vi "Auto.vi"() -> ()   [LabVIEW 2020]
uses:
  <vilib>/Utility/miscctls.llb/LVRowAndColumnTypeDef.ctl
  Global_Variable/A131258.vi
  Global_Variable/Global.vi
  Database/Global1.vi
  <userlib>/_MGI/1D Array/MGI Running Average/MGI Running Average(DBL).vi
  <vilib>/addons/database/Connection.llb/DB Tools Open Connec (String).vi
  <vilib>/addons/database/Connection.llb/Conn Execute.vi
  <vilib>/addons/database/Recordset.llb/Rec Fetch Recordset Data (R).vi
  Libraries/S7/S7.lvlib
  <vilib>/addons/database/NI_Database_API.lvlib
panel:
  out "左工位":cluster{dbl[], dbl[]}[](graph)
  in  "判定结果 2":bool[][](array[boolean])=[[TRUE]]
  out "STEP 4":string
  out "STEP 3":string
  in  "STEP 2":string
  out "右code 2":string
  in  "Initialize 7":bool
  in  "Initialize 6":bool
  out "初始化 2":bool[](array[boolean])
  out "左code":string
  out "右工位":cluster{dbl[], dbl[]}[](graph)
  in  "Initialize 4":bool
  in  "Initialize 2":bool
  out "初始化":bool[](array[boolean])
  in  "判定结果":bool[][](array[boolean])=[[TRUE]]
  in  "STEP":string
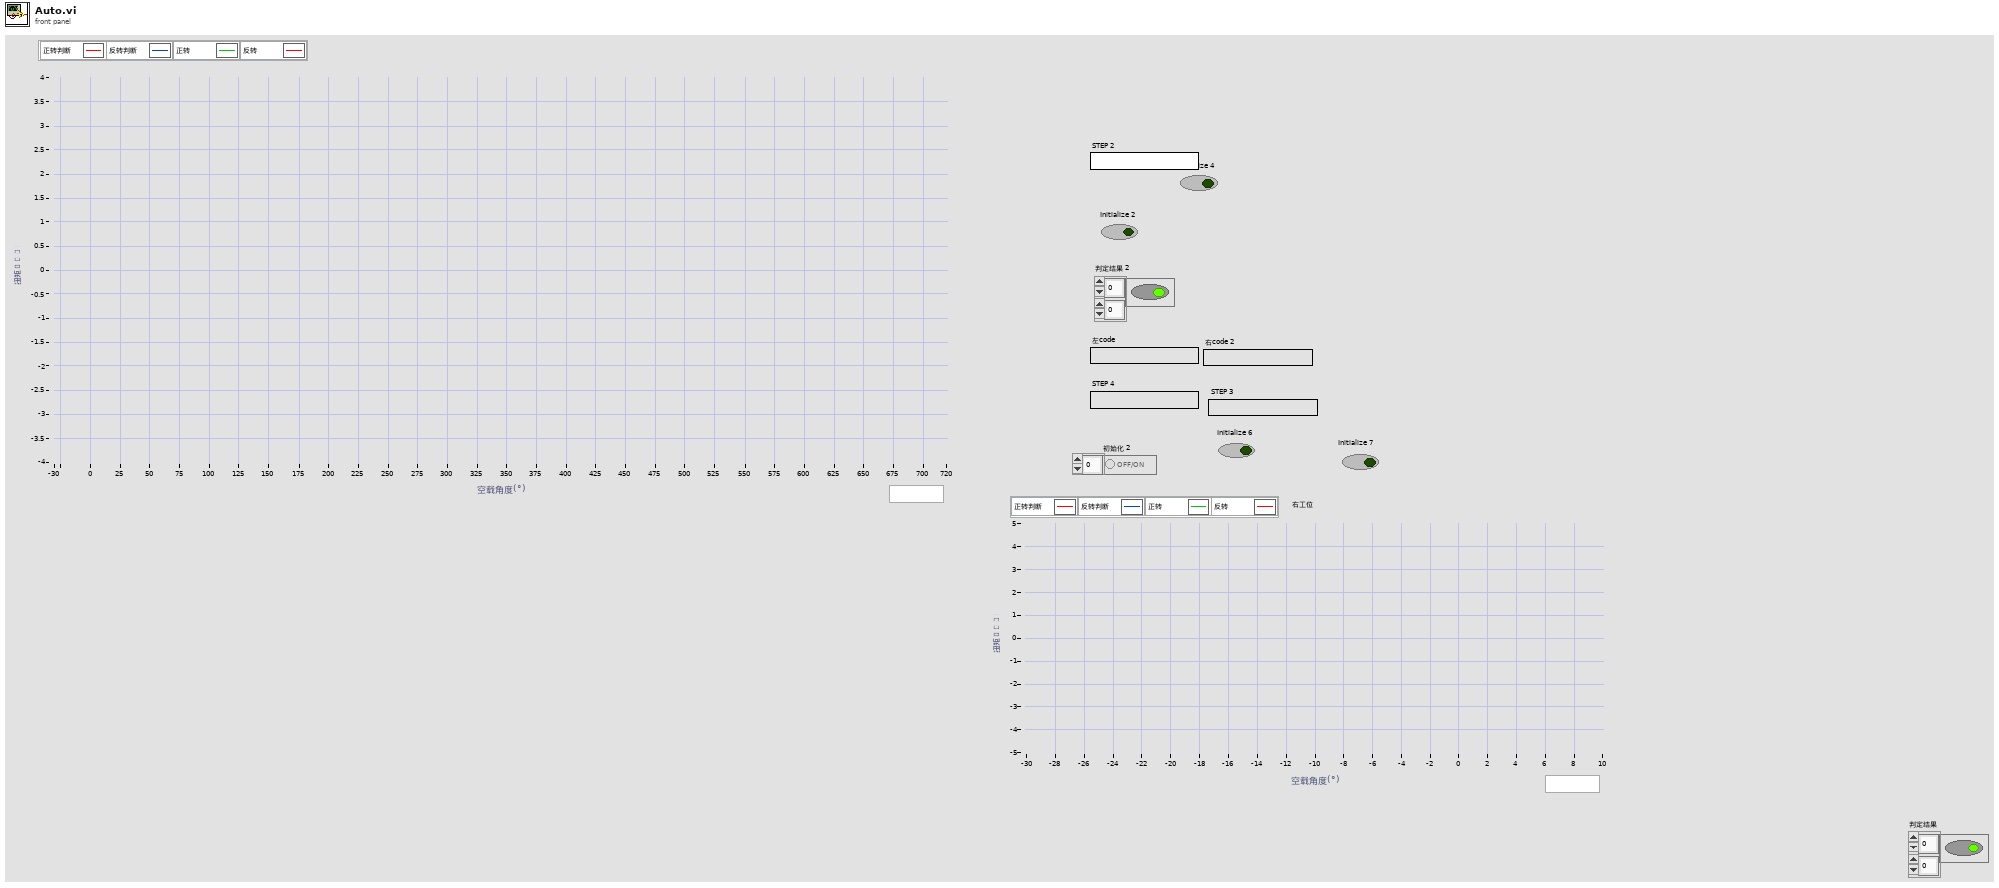
[diagram p1: front panel]
types:
  T1 = enum32{"Invalid", "Standard", "Closed", "Hidden", "Minimized", "Maximized"}
  T2 = typedef "LVRowAndColumnTypeDef.ctl" = cluster{"Row":i32, "Column":i32}
  T3 = typedef "lveventtype.ctl" = enum32{"Null", "Timeout", "Annotation Menu Selection", "Annotation Menu Selection?", "App Instance Close", "App Instance Close?", "Autoscale Range Change", "Bookmark Info Change", "Cell Edit", "Cell Edit?", "Cursor Grab", "Cursor Grab?", "Cursor Menu Selection", "Cursor Menu Selection?", "Cursor Move", "Cursor Release", "Data Change", "Direction Change", "Display State Change", "Drag Ended", "Drag Enter", "Drag Leave", "Drag Over", "Drag Source Update", "Drag Starting", "Drag Starting?", "Drop", "Exec State Change", "Key Down", "Key Down?", "Key Repeat", "Key Repeat?", "Key Up", "Listbox Double Click", "Menu Activation?", "Menu Selection (App)", "Menu Selection? (App)", "Menu Selection (User)", "Mouse Down", "Mouse Down?", "Mouse Enter", "Mouse Leave", "Mouse Move", "Mouse Up", "Mouse Wheel", "NI Security User Change (App)", "Pane Size", "Panel Close", "Panel Close?", "Panel Resize", "Plot Attribute Change", "Scale Range Change", "Shortcut Menu Activation?", "Shortcut Menu Selection (App)", "Shortcut Menu Selection? (App)", "Shortcut Menu Selection (User)", "Tree Double Click", "Tree Drag", "Tree Drag?", "Tree Drop", "Tree Drop?", "Tree Item Close", "Tree Item Close?", "Tree Item Open", "Tree Item Open?", "User Event", "Value Change"}
  T4 = typedef "LVPoint32TypeDef.ctl" = cluster{"Horizontal":i32, "Vertical":i32}
  T5 = cluster{"扭矩判定":cluster{"单位":string, "下限":dbl, "上限":dbl}, "正转扭矩最大值":cluster{"单位":string, "下限":dbl, "上限":dbl}, "正转扭矩最小值":cluster{"单位":string, "下限":dbl, "上限":dbl}, "正转扭矩波动值":cluster{"单位":string, "下限":dbl, "上限":dbl}, "正转平均扭矩值":cluster{"单位":string, "下限":dbl, "上限":dbl}, "反转扭矩最大值":cluster{"单位":string, "下限":dbl, "上限":dbl}, "反转扭矩最小值":cluster{"单位":string, "下限":dbl, "上限":dbl}, "反转扭矩波动值":cluster{"单位":string, "下限":dbl, "上限":dbl}, "反转扭矩平均值":cluster{"单位":string, "下限":dbl, "上限":dbl}, "正/逆转平均扭矩差":cluster{"单位":string, "下限":dbl, "上限":dbl}}
  T6 = cluster{"正向判定X值":cluster{"单位":string, "下限":dbl, "上限":dbl}, "正向判定Y值":cluster{"单位":string, "下限":dbl, "上限":dbl}, "逆向判定X值":cluster{"单位":string, "下限":dbl, "上限":dbl}, "逆向判定Y值":cluster{"单位":string, "下限":dbl, "上限":dbl}}
  T7 = cluster{"左平均扭矩":cluster{"正转":dbl, "反转":dbl}, "左矩波动":cluster{"正转":dbl, "反转":dbl}, "左空载":cluster{"正转":dbl, "反转":dbl}, "右平均扭矩":cluster{"正转":dbl, "反转":dbl}, "右扭矩波动":cluster{"正转":dbl, "反转":dbl}, "右空载":cluster{"正转":dbl, "反转":dbl}, "扭矩对称":cluster{"左":dbl, "右":dbl}, "左零点漂移":cluster{"正":dbl, "反":dbl}, "右零点漂移":cluster{"正":dbl, "反":dbl}}
  T8 = typedef "NI_Database_API.lvlib/Conn ObjectReference.ctl" = refnum<k1>
  T9 = typedef "NI_Database_API.lvlib/Rec ObjectReference.ctl" = refnum<k1>
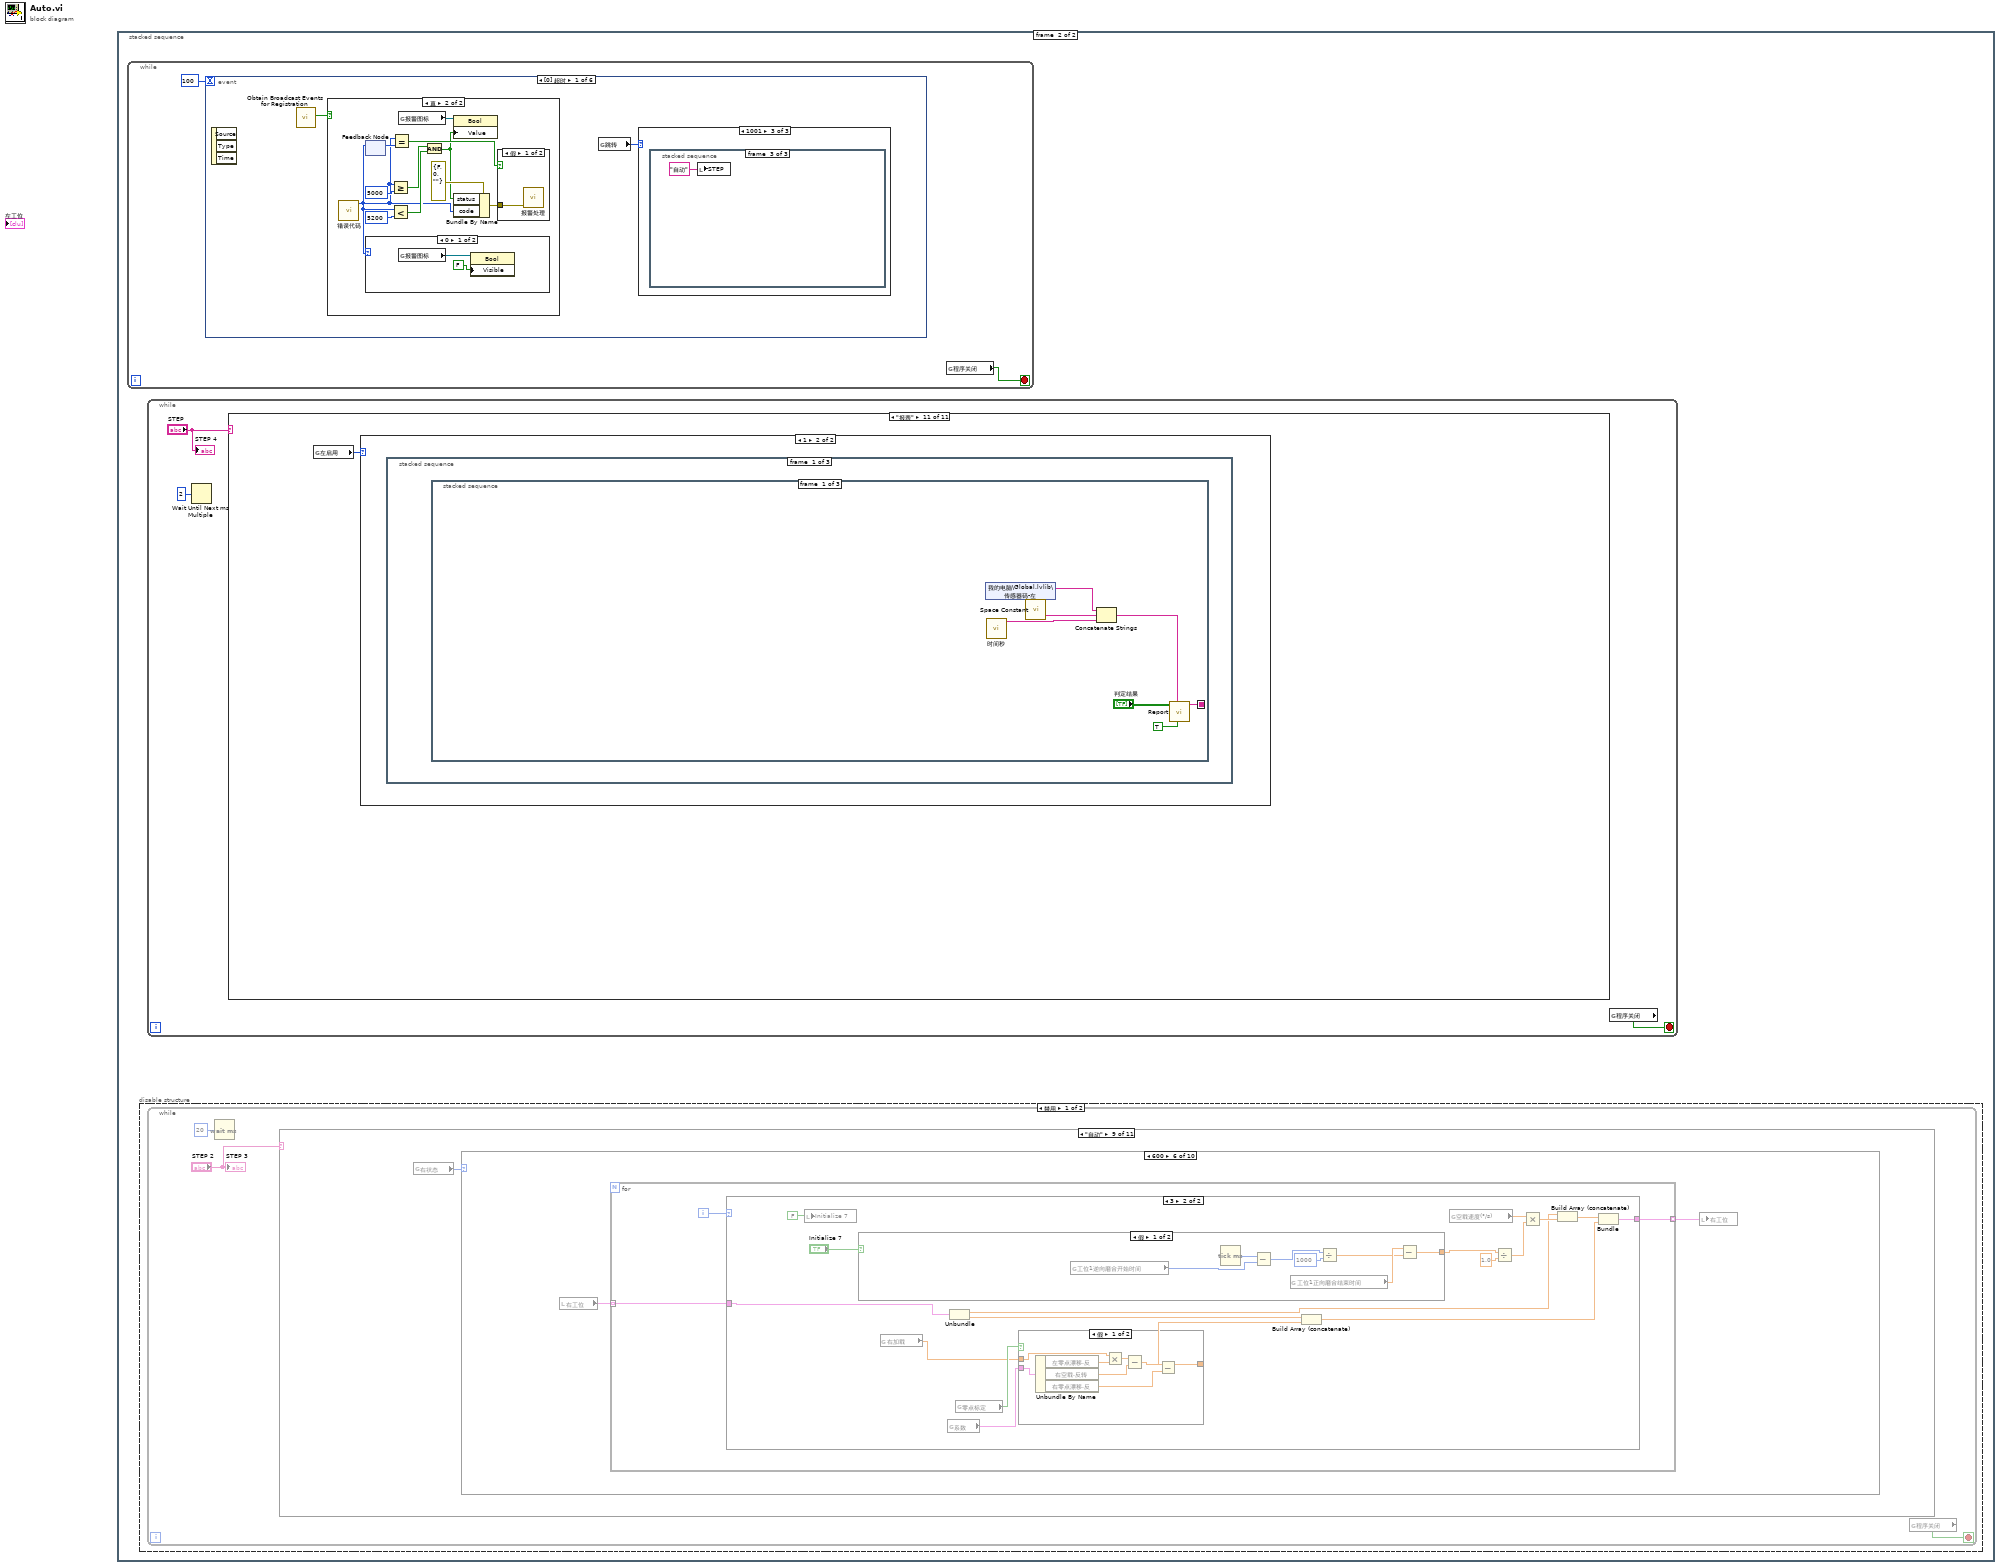
[diagram p0: block diagram]
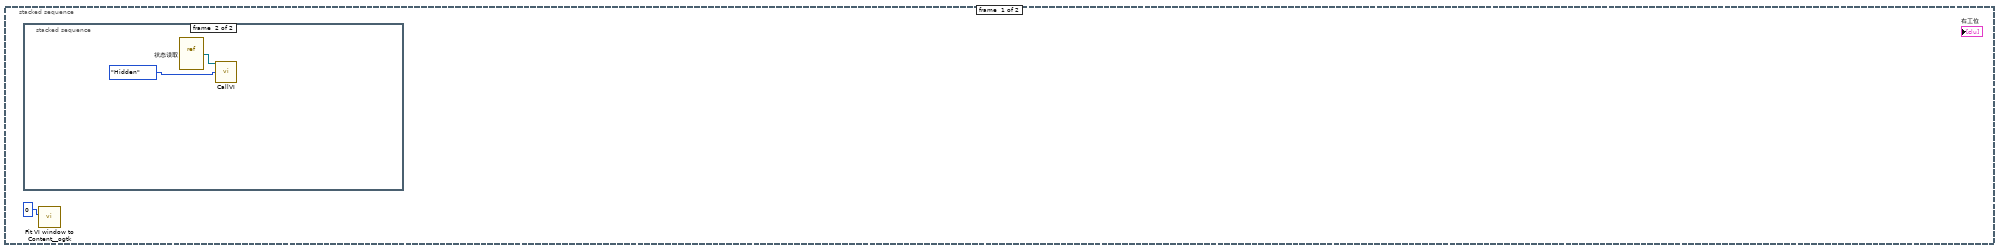
[diagram p2: hidden frame]
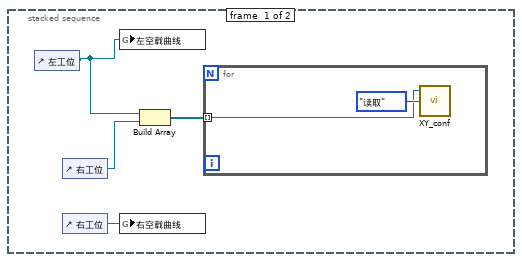
[diagram p3: hidden frame]
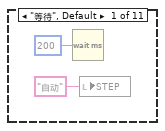
[diagram p4: hidden frame]
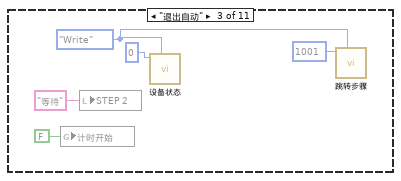
[diagram p6: hidden frame]
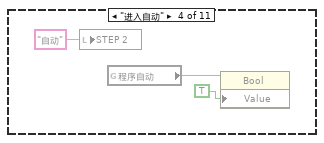
[diagram p7: hidden frame]
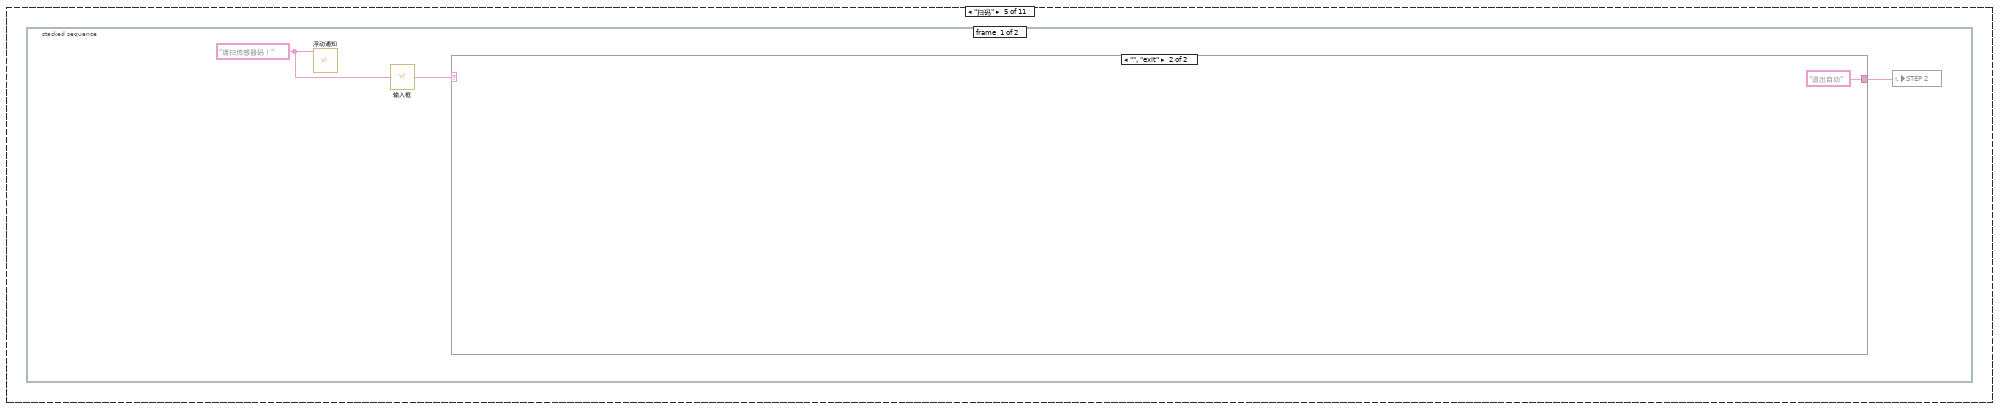
[diagram p8: hidden frame]
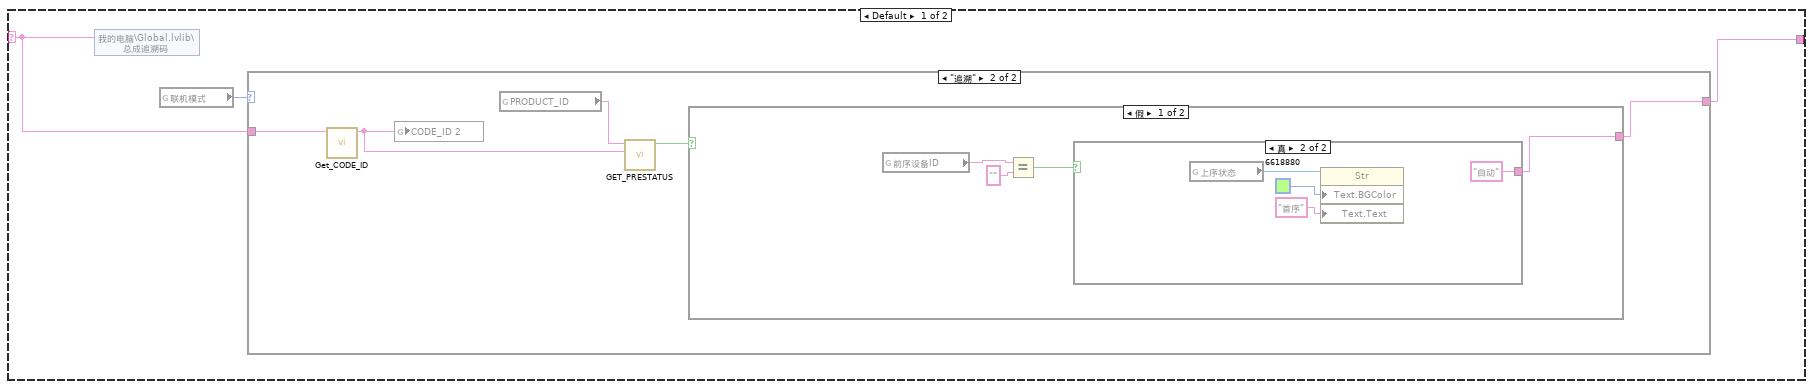
[diagram p9: hidden frame]
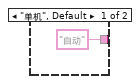
[diagram p10: hidden frame]
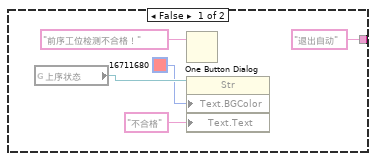
[diagram p11: hidden frame]
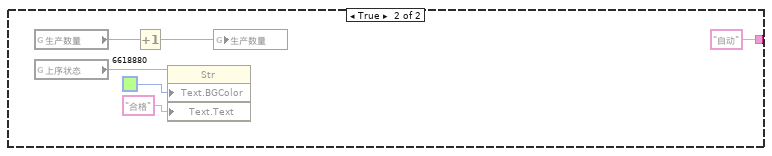
[diagram p12: hidden frame]
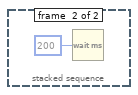
[diagram p13: hidden frame]
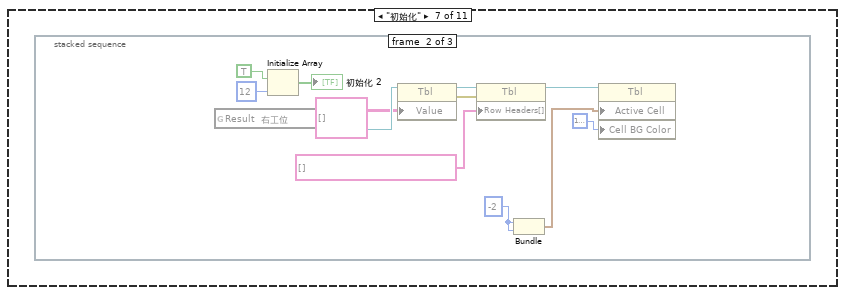
[diagram p15: hidden frame]
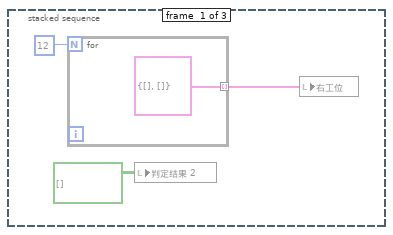
[diagram p16: hidden frame]
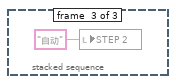
[diagram p17: hidden frame]
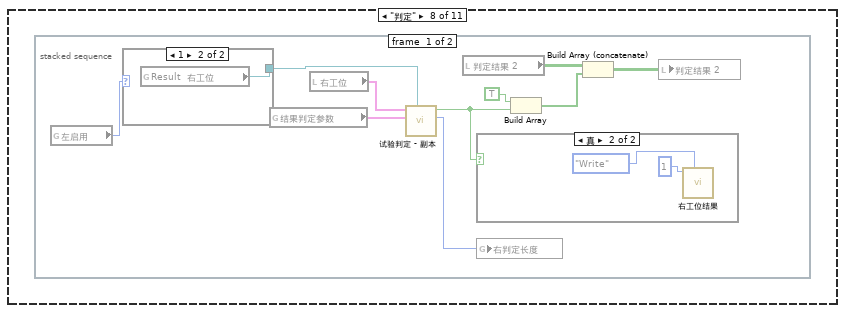
[diagram p18: hidden frame]
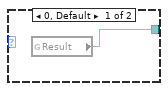
[diagram p19: hidden frame]
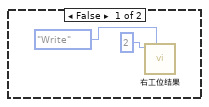
[diagram p20: hidden frame]
diagram:
  n1 = stacked-sequence {
    frame #0 {
      n2 = stacked-sequence {
        frame #0 {
          n3 = control-ref of="左工位"() -> (w2:refnum<vi>)
          n4 = control-ref of="右工位"() -> (w4:refnum<vi>)
          n5 = control-ref of="右工位"() -> (w5:refnum<vi>)
          n6 = global write "A131258.vi" "左空载曲线"(w2) -> ()
          n7 = global write "A131258.vi" "右空载曲线"(w5) -> ()
          n8 = Build Array(w2, w4) -> (w3:refnum<vi>[])
          n9 = for {
            tunnel: w3 -> [w6] mode=indexing
            n10 = call "XY_conf.vi"("方式"=enum16{"写入", "读取"}."读取", "XY图引用"=w6) -> ()  [unwired: 3 in, 1 out]
          }
        }
        frame #1 {
          n11 = vi-ref "状态读取.vi"() -> (w9:refnum<vi>)
          n12 = call "CallVI.vi"("VI引用"=w9, "状态"=T1."Hidden") -> ()  [unwired: 11 in, 3 out]
        }
      }
      n13 = call <userlib>:"Fit VI window to Content__ogtk.vi"("border spacing (2 px)"=0) -> ()  [unwired: 5 in, 2 out]
    }
    frame #1 {
      n14 = while {
        stop <- w728 stop-if-true
        n15 = event shown="[0] 超时" {
          selector: _ -> [_ _ _ _ _ _]
          dyn-events: _ -> [_ _ _ _ _ _]
          timeout: 100 -> [_ _ _ _ _ _]
          event Timeout {
            n16 = event-data() -> ()  [unwired: 1 in, 3 out]
            n17 = call "Obtain Broadcast Events for Registration.vi"() -> ("Already running?"=w731:bool)  [unwired: 9 in, 2 out]
            n18 = case shown="真" w731 {
              frame False {
                n19 = local write "STEP"("手动" ("STEP")) -> ()
              }
              frame True {
                n20 = call "错误代码.vi"() -> ("Status_Read"=w744:u32)  [unwired: 11 in]
                n21 = feedback #1() -> (w754:u32)  [unwired: 1 in]
                n22 = feedback-in #1(w744) -> ()
                n23 = case shown="0" w744 {
                  frame 0 {
                    n24 = global read "Global.vi" "报警图标"() -> (w755:refnum<vi>)
                    n25 = property class="Bool"(reference=w755, "Visible"=FALSE ("可见")) -> ()  [unwired: 1 in, 2 out]
                  }
                  frame 1, Default {
                    n26 = global read "Global.vi" "报警图标"() -> (w758:refnum<vi>)
                    n27 = property class="Bool"(reference=w758, "Visible"=TRUE ("可见")) -> ()  [unwired: 1 in, 2 out]
                  }
                }
                n28 = Greater Or Equal?(x=w744, y=i16 5000) -> (x >= y?=w752:bool)
                n29 = Less?(x=w744, y=i16 5200) -> (x < y?=w753:bool)
                n30 = Equal?(x=w744, y=w754) -> (x = y?=w751:bool)
                n31 = global read "Global.vi" "报警图标"() -> (w746:refnum<vi>)
                n32 = And(x=w752, y=w753) -> (x .and. y?=w745:bool)
                n33 = property class="Bool"(reference=w746, "Value"=w745) -> ()  [unwired: 1 in, 2 out]
                n34 = Bundle By Name(cluster=errorcluster {"status"=FALSE, "code"=0, "source"=""} ("错误常量"), "status"=w745, "code"=w744) -> (w750:errorcluster)
                n35 = case shown="假" w751 {
                  tunnel: w750 -> [w759 _]
                  frame False {
                    n36 = call "报警处理.vi"("错误常量"=w759) -> ()  [unwired: 9 in, 2 out]
                  }
                  frame True {
                  }
                }
              }
            }
            n37 = global read "Global.vi" "跳转"() -> (w730:i16)
            n38 = case shown="1001" w730 {
              frame 0, Default {
              }
              frame 1000 {
                n39 = stacked-sequence {
                  frame #0 {
                    w732 = "" ("文本.文本")
                    n40 = Wait (ms)(milliseconds to wait=u32 200 ("等待时间（毫秒）")) -> ()  [unwired: 1 out]
                    n41 = shared-variable "我的电脑\\Global.lvlib\\传感器码-右"(w732) -> ()  [unwired: 1 in, 1 out]
                    n42 = shared-variable "我的电脑\\Global.lvlib\\传感器码-左"(w732) -> ()  [unwired: 1 in, 1 out]
                    n43 = call "跳转步骤.vi"("枚举"=enum16{"Read", "Write"}."Write", "Status_Write"=u16 1001 ("跳转步骤")) -> ()  [unwired: 9 in, 1 out]
                  }
                  frame #1 {
                    n44 = local write "STEP"("扫码" ("STEP")) -> ()
                  }
                }
              }
              frame 1001 {
                n45 = stacked-sequence {
                  frame #0 {
                    n46 = Wait (ms)(milliseconds to wait=u32 100 ("等待时间（毫秒）")) -> ()  [unwired: 1 out]
                  }
                  frame #1 {
                    n47 = global read "Global.vi" "左在位"() -> (w738:i16)
                    n48 = case shown="1" w738 {
                      frame 0, Default {
                      }
                      frame 1 {
                        w740 = enum16{"Read", "Write"}."Write" ("枚举")
                        n49 = call "左工位在位.vi"("枚举"=w740, "Status_Write"=u16 0 ("左工位工件在位")) -> ()  [unwired: 9 in, 1 out]
                        n50 = call "左工位状态.vi"("枚举"=w740, "Status_Write"=u16 1001 ("左工位状态")) -> ()  [unwired: 9 in, 1 out]
                      }
                    }
                  }
                  frame #2 {
                    n51 = local write "STEP"("自动" ("STEP")) -> ()
                  }
                }
              }
            }
          }
          event Menu Selection (User) {
            n52 = event-data() -> ("ItemTag"=w760:string)  [unwired: 1 in, 2 out]
            n53 = case shown="\"真\"" w760 {
              frame "假", Default {
              }
              frame "真" {
              }
            }
          }
          event "右工位", "左工位": Scale Range Change {
            n54 = event-data() -> ("CtlRef"=w761:refnum<vi>)  [unwired: 1 in]
            n55 = call "XY_conf.vi"("方式"=enum16{"写入", "读取"}."写入", "XY图引用"=w761) -> ()  [unwired: 3 in, 1 out]
          }
          event Panel Close {
            n56 = event-data() -> ()  [unwired: 1 in, 4 out]
            n57 = global write "Global.vi" "程序关闭"(TRUE ("程序关闭")) -> ()
          }
          event "右工位", "左工位": Mouse Enter; "右工位", "左工位": Mouse Leave; "右工位": Cursor Move; "左工位": Mouse Move {
            n58 = event-data() -> ("CtlRef"=w766:refnum<vi>, "Type"=w765:T3)  [unwired: 1 in]
            n59 = call "CursorShow.vi"("nameShow"=TRUE, "Type"=w765, "Graph"=w766) -> ()  [unwired: 7 in, 2 out]
          }
          event "右工位", "左工位": Mouse Down {
            n60 = event-data() -> ("CtlRef"=w771:refnum<vi>, "Coords"=w770:T4, "Type"=w769:T3)  [unwired: 1 in]
            n61 = invoke class="XYGraph (严格)" method="Map Coords To XY"(reference=w771, "Coords"=w770) -> (reference out=w768:refnum<vi>, "XY"=w767:cluster{"X":dbl, "Y":dbl})  [unwired: 5 in, 5 out]
            n62 = call "CursorShow.vi"("游标.游标位置"=w767, "Type"=w769, "Graph"=w768) -> ()  [unwired: 7 in, 2 out]
          }
        }
        n63 = global read "Global.vi" "程序关闭"() -> (w728:bool)
      }
      n64 = disable-structure shown="禁用" {
        frame Disabled {
          n65 = while {
            stop <- w12 stop-if-true
            n66 = Wait (ms)(milliseconds to wait=u32 20 ("等待时间（毫秒）")) -> ()  [unwired: 1 out]
            n67 = case shown="\"自动\"" "STEP 2" {
              frame "等待", Default {
                n68 = Wait (ms)(milliseconds to wait=u32 200 ("等待时间（毫秒）")) -> ()  [unwired: 1 out]
                n69 = local write "STEP"("自动" ("STEP")) -> ()
              }
              frame "手动" {
              }
              frame "退出自动" {
                w16 = enum16{"Read", "Write"}."Write" ("枚举")
                n70 = global write "Global.vi" "计时开始"(FALSE ("计时开始")) -> ()
                n71 = local write "STEP 2"("等待" ("STEP")) -> ()
                n72 = call "设备状态.vi"("枚举"=w16, "Status_Write"=i16 0) -> ()  [unwired: 9 in, 1 out]
                n73 = call "跳转步骤.vi"("枚举"=w16, "Status_Write"=i16 1001) -> ()  [unwired: 9 in, 1 out]
              }
              frame "进入自动" {
                n74 = local write "STEP 2"("自动" ("STEP")) -> ()
                n75 = global read "Global.vi" "程序自动"() -> (w21:refnum<vi>)
                n76 = property class="Bool"(reference=w21, "Value"=TRUE) -> ()  [unwired: 1 in, 2 out]
              }
              frame "扫码" {
                n77 = stacked-sequence {
                  frame #0 {
                    w24 = "请扫传感器码！" ("提示信息")
                    n78 = call "浮动通知.vi"("通知内容"=w24) -> ()  [unwired: 11 in]
                    n79 = call "输入框.vi"("提示信息"=w24) -> ("条形码输出"=w25:string)
                    n80 = case shown="\"\", \"exit\"" w25 {
                      selector: w25 -> [w26 _]
                      tunnel: [w28 "退出自动" ("State(s) in Front (\"\")")] -> w23
                      frame Default {
                        n81 = shared-variable "我的电脑\\Global.lvlib\\总成追溯码"(w26) -> ()  [unwired: 1 in, 1 out]
                        n82 = global read "Global1.vi" "联机模式"() -> (w27:enum16{"单机", "追溯"})
                        n83 = case shown="\"追溯\"" w27 {
                          tunnel: ["自动" ("State(s) in Front (\"\")") w34] -> w28
                          tunnel: w26 -> [_ w33]
                          frame "单机", Default {
                          }
                          frame "追溯" {
                            n84 = call "Get_CODE_ID.vi"("CODE_MAIN"=w33) -> ("CODE_ID"=w30:string)  [unwired: 10 in]
                            n85 = global write "追溯Global.vi" "CODE_ID 2"(w30) -> ()
                            n86 = global read "追溯Global.vi" "PRODUCT_ID"() -> (w32:string)
                            n87 = call "GET_PRESTATUS.vi"("CODE_ID"=w30, "PRODUCT_ID"=w32) -> ("OK?"=w31:bool)  [unwired: 8 in, 1 out]
                            n88 = case shown="假" w31 {
                              tunnel: [w38 "自动" ("State(s) in Front (\"\")")] -> w34
                              frame False {
                                n89 = global read "追溯Global.vi" "前序设备ID"() -> (w37:string)
                                n90 = Equal?(x=w37, y="") -> (x = y?=w36:bool)
                                n91 = case shown="真" w36 {
                                tunnel: ["退出自动" ("State(s) in Front (\"\")") "自动" ("State(s) in Front (\"\")")] -> w38
                                frame False {
                                n92 = global read "Global.vi" "上序状态"() -> (w41:refnum<vi>)
                                n93 = One Button Dialog(message="前序工位检测不合格！" ("消息")) -> ()  [unwired: 1 in, 1 out]
                                n94 = property class="Str"(reference=w41, "Text.BGColor"=u32 16711680 ("文本.文本颜色:背景色"), "Text.Text"="不合格" ("文本.文本")) -> ()  [unwired: 1 in, 2 out]
                                }
                                frame True {
                                n95 = global read "Global.vi" "上序状态"() -> (w46:refnum<vi>)
                                n96 = property class="Str"(reference=w46, "Text.BGColor"=u32 6618880 ("文本.文本颜色:背景色"), "Text.Text"="首序" ("文本.文本")) -> ()  [unwired: 1 in, 2 out]
                                }
                                }
                              }
                              frame True {
                                n97 = global read "Global.vi" "生产数量"() -> (w51:i32)
                                n98 = global read "Global.vi" "上序状态"() -> (w50:refnum<vi>)
                                n99 = Increment(x=w51) -> (x+1=w52:i32)
                                n100 = property class="Str"(reference=w50, "Text.BGColor"=u32 6618880 ("文本.文本颜色:背景色"), "Text.Text"="合格" ("文本.文本")) -> ()  [unwired: 1 in, 2 out]
                                n101 = global write "Global.vi" "生产数量"(w52) -> ()
                              }
                            }
                          }
                        }
                      }
                      frame "", "exit" {
                      }
                    }
                    n102 = local write "STEP 2"(w23) -> ()
                  }
                  frame #1 {
                    n103 = Wait (ms)(milliseconds to wait=u32 200 ("等待时间（毫秒）")) -> ()  [unwired: 1 out]
                  }
                }
              }
              frame "工位判断" {
              }
              frame "初始化" {
                n104 = stacked-sequence {
                  frame #0 {
                    n105 = for {
                      N: 12 -> [_]
                      tunnel: [cluster{dbl[], dbl[]} {[], []}] -> w57 mode=indexing
                    }
                    n106 = local write "判定结果 2"(bool[][] [] ("判定结果")) -> ()
                    n107 = local write "右工位"(w57) -> ()
                  }
                  frame #1 {
                    w60 = -2 ("维数大小")
                    n108 = global read "Global.vi" "Result  右工位"() -> (w69:refnum<vi>)
                    n109 = Initialize Array(TRUE, 12 ("维数大小")) -> (→"初始化 2":bool[])
                    n110 = property class="Tbl"(reference=w69, "Value"=string[][] []) -> (reference out=w70:refnum<vi>, error out=w71:errorcluster)  [unwired: 1 in]
                    n111 = property class="Tbl"(reference=w70, error in=w71, "Row Headers[]"=string[] [] ("列首字符串[]")) -> (reference out=w63:refnum<vi>)  [unwired: 1 out]
                    n112 = Bundle("维数大小"=w60, "维数大小"=w60) -> (w61:cluster{"维数大小":i32, "维数大小":i32})  [unwired: 1 in]
                    n113 = property class="Tbl"(reference=w63, "Active Cell"=w61, "Cell BG Color"=u32 16777216 ("活动单元格:单元格背景色")) -> ()  [unwired: 1 in, 2 out]
                  }
                  frame #2 {
                    n114 = local write "STEP 2"("自动" ("STEP")) -> ()
                  }
                }
              }
              frame "判定" {
                n115 = stacked-sequence {
                  frame #0 {
                    n116 = global read "Global.vi" "左启用"() -> (w73:i16)
                    n117 = case shown="1" w73 {
                      tunnel: [w83 w84] -> w80
                      frame 0, Default {
                        n118 = global read "Global.vi" "Result"() -> (w83:refnum<vi>)
                      }
                      frame 1 {
                        n119 = global read "Global.vi" "Result  右工位"() -> (w84:refnum<vi>)
                      }
                    }
                    n120 = global read "A131258.vi" "结果判定参数"() -> (w78:T5)
                    n121 = local read "右工位"() -> (w79:cluster{dbl[], dbl[]}[])
                    n122 = call "试验判定 - 副本.vi"("Result"=w80, "判定参数"=w78, "XY曲线"=w79) -> ("判定项长度"=w77:i32, "OK？"=w81:bool)  [unwired: 7 in]
                    n123 = local read "判定结果 2"() -> (w76:bool[][])
                    n124 = case shown="真" w81 {
                      frame False {
                        n125 = call "右工位结果.vi"("枚举"=enum16{"Read", "Write"}."Write", "Status_Write"=u16 2 ("左工位生产结果")) -> ()  [unwired: 9 in, 1 out]
                      }
                      frame True {
                        n126 = call "右工位结果.vi"("枚举"=enum16{"Read", "Write"}."Write", "Status_Write"=u16 1 ("左工位生产结果")) -> ()  [unwired: 9 in, 1 out]
                      }
                    }
                    n127 = global write "判定参数.vi" "右判定长度"(w77) -> ()
                    n128 = Build Array(TRUE ("元素"), w81) -> (w74:bool[])
                    n129 = Build Array (concatenate)(w76, w74) -> (w75:bool[][])
                    n130 = local write "判定结果 2"(w75) -> ()
                  }
                  frame #1 {
                    n131 = local write "STEP 2"("报表" ("STEP")) -> ()
                  }
                }
              }
              frame "自动" {
                n132 = global read "Global.vi" "右状态"() -> (w90:i16)
                n133 = case shown="600" w90 {
                  frame 0, Default {
                  }
                  frame 1 {
                  }
                  frame 3 {
                    n134 = stacked-sequence {
                      frame #0 {
                        n135 = call "右工位结果.vi"("枚举"=enum16{"Read", "Write"}."Write", "Status_Write"=i16 0) -> ()  [unwired: 9 in, 1 out]
                        n136 = local write "判定结果 2"(bool[][] [] ("判定结果")) -> ()
                      }
                      frame #1 {
                        n137 = global read "Global.vi" "空载速度(°/s) 2"() -> (w94:sgl)
                        n138 = Multiply(x=w94, y=sgl 6.0) -> (x*y=w95:sgl)
                        n139 = global write "Global.vi" "空载速度(°/s)"(w95) -> ()
                      }
                    }
                  }
                  frame 200 {
                    n140 = stacked-sequence {
                      frame #0 {
                        w97 = TRUE ("Initialize 2")
                        n141 = local write "Initialize 7"(w97) -> ()
                        n142 = local write "Initialize 6"(w97) -> ()
                        n143 = call "右工位结果.vi"("枚举"=enum16{"Read", "Write"}."Write", "Status_Write"=u16 0 ("左工位生产结果")) -> ()  [unwired: 9 in, 1 out]
                      }
                      frame #1 {
                        n144 = local read "右工位"() -> (w100:cluster{dbl[], dbl[]}[])
                        n145 = for {
                          tunnel: [w103] -> w101 mode=indexing
                          tunnel: w100 -> [w102] mode=indexing
                          i -> [w104]
                          n146 = case shown="0" w104 {
                            tunnel: [w105 w106 w114] -> w103
                            tunnel: w102 -> [w105 _ _]
                            frame Default {
                            }
                            frame 0 {
                              n147 = global read "A131258.vi" "判定框参数"() -> (w111:T6)
                              n148 = Unbundle By Name(w111) -> ("正向判定X值.下限"=w110:dbl, "正向判定X值.上限"=w109:dbl, "正向判定Y值.下限"=w108:dbl, "正向判定Y值.上限"=w107:dbl)
                              n149 = Build Array(w109, w109, w110, w110, w109) -> (w113:dbl[])
                              n150 = Build Array(w107, w108, w108, w107, w107) -> (w112:dbl[])
                              n151 = Bundle(w113, w112) -> (w106:cluster{dbl[], dbl[]})  [unwired: 1 in]
                            }
                            frame 1 {
                              n152 = global read "A131258.vi" "判定框参数"() -> (w119:T6)
                              n153 = Unbundle By Name(w119) -> ("逆向判定X值.下限"=w118:dbl, "逆向判定X值.上限"=w117:dbl, "逆向判定Y值.下限"=w116:dbl, "逆向判定Y值.上限"=w115:dbl)
                              n154 = Build Array(w117, w117, w118, w118, w117) -> (w121:dbl[])
                              n155 = Build Array(w115, w116, w116, w115, w115) -> (w120:dbl[])
                              n156 = Bundle(w121, w120) -> (w114:cluster{dbl[], dbl[]})  [unwired: 1 in]
                            }
                          }
                        }
                        n157 = local write "右工位"(w101) -> ()
                      }
                    }
                  }
                  frame 500 {
                    n158 = local read "右工位"() -> (w123:cluster{dbl[], dbl[]}[])
                    n159 = for {
                      tunnel: w123 -> [w125] mode=indexing
                      tunnel: [w124] -> w122 mode=indexing
                      i -> [w126]
                      n160 = case shown="2" w126 {
                        tunnel: w125 -> [w127 w144]
                        tunnel: [w127 w136] -> w124
                        frame Default {
                        }
                        frame 2 {
                          n161 = local write "Initialize 6"(FALSE ("Initialize 2")) -> ()
                          n162 = case shown="假" "Initialize 6" {
                            tunnel: [w157 0.0] -> w141
                            frame False {
                              n163 = global read "全局 1.vi" "工位1正向磨合开始时间"() -> (w161:u32)
                              n164 = Tick Count (ms)() -> (millisecond timer value=w160:u32)
                              n165 = Subtract(x=w160, y=w161) -> (x-y=w159:u32)
                              n166 = Divide(x=w159, y=u32 1000) -> (x/y=w157:dbl)
                              n167 = global write "全局 1.vi" "工位1正向磨合结束时间"(w157) -> ()
                            }
                            frame True {
                              n168 = Tick Count (ms)() -> (millisecond timer value=w162:u32)
                              n169 = global write "全局 1.vi" "工位1正向磨合开始时间"(w162) -> ()
                            }
                          }
                          n170 = global read "全局2.vi" "右加载"() -> (w129:dbl)
                          n171 = global read "A131258.vi" "零点标定"() -> (w131:bool)
                          n172 = global read "A131258.vi" "系数"() -> (w130:T7)
                          n173 = Unbundle(w144) -> (w138:dbl[], w143:dbl[])
                          n174 = case shown="假" w131 {
                            tunnel: [w146 w153] -> w128
                            tunnel: w130 -> [w152 w156]
                            tunnel: w129 -> [w151 w155]
                            frame False {
                              n175 = Unbundle By Name(w152) -> ("左零点漂移.正"=w150:dbl, "右空载.正转"=w147:dbl, "右零点漂移.正"=w145:dbl)
                              n176 = Multiply(x=w151, y=w150) -> (x*y=w148:dbl)
                              n177 = Subtract(x=w148, y=w147) -> (x-y=w149:dbl)
                              n178 = Subtract(x=w149, y=w145) -> (x-y=w146:dbl)
                            }
                            frame True {
                              n179 = Unbundle By Name(w156) -> ("右零点漂移.正"=w154:dbl)
                              n180 = Subtract(x=w155, y=w154) -> (x-y=w153:dbl)
                            }
                          }
                          n181 = Build Array (concatenate)(w143, w128) -> (w135:dbl[])
                          n182 = global read "Global.vi" "空载速度(°/s)"() -> (w140:sgl)
                          n183 = Divide(x=w141, y=1.0) -> (x/y=w133:dbl)
                          n184 = Multiply(x=w140, y=w133) -> (x*y=w139:dbl)
                          n185 = Build Array (concatenate)(w138, w139) -> (w137:dbl[])
                          n186 = Bundle(w137, w135) -> (w136:cluster{dbl[], dbl[]})  [unwired: 1 in]
                        }
                      }
                    }
                    n187 = local write "右工位"(w122) -> ()
                  }
                  frame 600 {
                    n188 = local read "右工位"() -> (w165:cluster{dbl[], dbl[]}[])
                    n189 = for {
                      tunnel: w165 -> [w167] mode=indexing
                      tunnel: [w166] -> w164 mode=indexing
                      i -> [w168]
                      n190 = case shown="3" w168 {
                        tunnel: w167 -> [w169 w186]
                        tunnel: [w169 w178] -> w166
                        frame 0, Default {
                        }
                        frame 3 {
                          n191 = local write "Initialize 7"(FALSE ("Initialize 2")) -> ()
                          n192 = case shown="假" "Initialize 7" {
                            tunnel: [w199 w206] -> w175
                            frame False {
                              n193 = global read "全局 1.vi" "工位1逆向磨合开始时间"() -> (w205:u32)
                              n194 = Tick Count (ms)() -> (millisecond timer value=w204:u32)
                              n195 = Subtract(x=w204, y=w205) -> (x-y=w203:u32)
                              n196 = global read "全局 1.vi" "工位1正向磨合结束时间"() -> (w201:dbl)
                              n197 = Divide(x=w203, y=u32 1000) -> (x/y=w200:dbl)
                              n198 = Subtract(x=w201, y=w200) -> (x-y=w199:dbl)
                            }
                            frame True {
                              n199 = Tick Count (ms)() -> (millisecond timer value=w207:u32)
                              n200 = global write "全局 1.vi" "工位1逆向磨合开始时间"(w207) -> ()
                              n201 = global read "全局 1.vi" "工位1正向磨合结束时间"() -> (w206:dbl)
                            }
                          }
                          n202 = global read "全局2.vi" "右加载"() -> (w171:dbl)
                          n203 = global read "A131258.vi" "系数"() -> (w172:T7)
                          n204 = Unbundle(w186) -> (w181:dbl[], w185:dbl[])
                          n205 = global read "A131258.vi" "零点标定"() -> (w173:bool)
                          n206 = case shown="假" w173 {
                            tunnel: [w188 w195] -> w170
                            tunnel: w172 -> [w194 w198]
                            tunnel: w171 -> [w193 w197]
                            frame False {
                              n207 = Unbundle By Name(w194) -> ("左零点漂移.反"=w192:dbl, "右空载.反转"=w189:dbl, "右零点漂移.反"=w187:dbl)
                              n208 = Multiply(x=w193, y=w192) -> (x*y=w190:dbl)
                              n209 = Subtract(x=w190, y=w189) -> (x-y=w191:dbl)
                              n210 = Subtract(x=w191, y=w187) -> (x-y=w188:dbl)
                            }
                            frame True {
                              n211 = Unbundle By Name(w198) -> ("右零点漂移.反"=w196:dbl)
                              n212 = Subtract(x=w197, y=w196) -> (x-y=w195:dbl)
                            }
                          }
                          n213 = Build Array (concatenate)(w185, w170) -> (w179:dbl[])
                          n214 = global read "Global.vi" "空载速度(°/s)"() -> (w183:sgl)
                          n215 = Divide(x=w175, y=1.0) -> (x/y=w176:dbl)
                          n216 = Multiply(x=w183, y=w176) -> (x*y=w182:dbl)
                          n217 = Build Array (concatenate)(w181, w182) -> (w180:dbl[])
                          n218 = Bundle(w180, w179) -> (w178:cluster{dbl[], dbl[]})  [unwired: 1 in]
                        }
                      }
                    }
                    n219 = local write "右工位"(w164) -> ()
                  }
                  frame 680 {
                    n220 = stacked-sequence {
                      frame #0 {
                        n221 = Wait (ms)(milliseconds to wait=u32 5 ("等待时间（毫秒）")) -> ()  [unwired: 1 out]
                      }
                      frame #1 {
                        n222 = local write "STEP 2"("判定" ("STEP")) -> ()
                      }
                    }
                  }
                  frame 730 {
                  }
                  frame 1001 {
                    n223 = stacked-sequence {
                      frame #0 {
                        n224 = Wait (ms)(milliseconds to wait=u32 50 ("等待时间（毫秒）")) -> ()  [unwired: 1 out]
                        n225 = shared-variable "我的电脑\\Global.lvlib\\工位追溯码"() -> (w210:string)  [unwired: 1 in, 1 out]
                        n226 = shared-variable "我的电脑\\Global.lvlib\\传感器码-右"(w210) -> ()  [unwired: 1 in, 1 out]
                      }
                      frame #1 {
                        n227 = global read "Global1.vi" "联机模式"() -> (w212:enum16{"单机", "追溯"})
                        n228 = case shown="\"追溯\"" w212 {
                          selector: w212 -> [_ w222]
                          frame "单机", Default {
                          }
                          frame "追溯" {
                            n229 = shared-variable "我的电脑\\Global.lvlib\\传感器码-右"() -> (w213:string)  [unwired: 1 in, 1 out]
                            n230 = global read "追溯Global.vi" "PRODUCT_ID"() -> (w219:string)
                            n231 = Bundle("String"=w213, "PRODUCT_ID"=w219) -> (w218:cluster{"String":string, "PRODUCT_ID":string})  [unwired: 1 in]
                            n232 = call "GetSQLstring.vi"("联机模式"=w222) -> ("错误输出"=w220:errorcluster, "连接字符串"=w221:string)  [unwired: 9 in]
                            n233 = call-poly <vilib>:"DB Tools Open Connection.vi"("error in (no error)"=w220, "connection information"=w221) -> ("error out"=w216:errorcluster, "connection reference"=w217:T8)  [unwired: 6 in]
                            n234 = Build Array(w218) -> (w214:cluster{"String":string, "PRODUCT_ID":string}[])
                            n235 = for {
                              tunnel: w217 -> [w230]
                              shift-right: [w227] -> w215
                              shift-left: w216 -> [w229]
                              tunnel: w214 -> [w223] mode=indexing
                              n236 = call <vilib>:"DB Tools Insert Data.vi"("data"=w223, "error in (no error)"=w229, "columns"=string[] ["CODE_SENSOR", "PRODUCT_ID"], "table"="Code", "connection reference"=w230) -> ("error out"=w228:errorcluster, "connection reference out"=w226:T8)  [unwired: 5 in]
                              n237 = case shown="错误 .." w228 {
                                selector: w228 -> [w232 w234]
                                tunnel: [w232 w235] -> w227
                                tunnel: [w231 w233] -> _
                                tunnel: w226 -> [w231 w233]
                                frame No Error {
                                }
                                frame Error {
                                n238 = call <vilib>:"Clear Errors.vi"("error in (no error)"=w234) -> ("error out"=w235:errorcluster)  [unwired: 5 in, 1 out]
                                }
                              }
                            }
                            n239 = call <vilib>:"Simple Error Handler.vi"("error in (no error)"=w215) -> ()  [unwired: 4 in, 5 out]
                          }
                        }
                      }
                      frame #2 {
                        n240 = global read "Global1.vi" "联机模式"() -> (w236:enum16{"单机", "追溯"})
                        n241 = case shown="\"追溯\"" w236 {
                          selector: w236 -> [_ w257]
                          frame "单机", Default {
                          }
                          frame "追溯" {
                            w249 = "'"
                            n242 = shared-variable "我的电脑\\Global.lvlib\\传感器码-右"() -> (w237:string)  [unwired: 1 in, 1 out]
                            n243 = global read "追溯Global.vi" "PRODUCT_ID"() -> (w250:string)
                            n244 = call "GetSQLstring.vi"("联机模式"=w257) -> ("错误输出"=w255:errorcluster, "连接字符串"=w256:string)  [unwired: 9 in]
                            n245 = Concatenate Strings("SELECT CODE_ID FROM CODE  WHERE CODE_SENSOR = '" ("table"), w237, w249, " AND PRODUCT_ID='" ("字符串"), w250, w249) -> (w248:string)
                            n246 = call-poly <vilib>:"DB Tools Open Connection.vi"("error in (no error)"=w255, "connection information"=w256) -> ("error out"=w254:errorcluster, "connection reference"=w253:T8)  [unwired: 6 in]
                            n247 = call-poly <vilib>:"DB Tools Execute Query.vi"("error in (no error)"=w254, "SQL query"=w248, "connection reference"=w253) -> ("error out"=w247:errorcluster, "recordset reference"=w246:T9)  [unwired: 5 in]
                            n248 = call-poly <vilib>:"DB Tools Fetch Recordset Data.vi"("error in (no error)"=w247, "recordset reference"=w246) -> ("error out"=w245:errorcluster, "recordset data"=w244:variant[][])  [unwired: 3 in, 1 out]
                            n249 = Variant To Data(error in=w245, type=string[][] [], Variant=w244) -> (data=w242:string[][])  [unwired: 1 out]
                            n250 = Index Array(array=w242, index (row)=0 ("索引 (行)")) -> (element=w241:string[])  [unwired: 1 in]
                            n251 = Index Array(array=w241, index=0 ("索引")) -> (element=→"右code 2":string)
                          }
                        }
                      }
                      frame #3 {
                        n252 = Wait (ms)(milliseconds to wait=u32 50 ("等待时间（毫秒）")) -> ()  [unwired: 1 out]
                        n253 = local write "STEP 2"("自动" ("STEP")) -> ()
                        n254 = call "右工位状态.vi"("枚举"=enum16{"Read", "Write"}."Write", "Status_Write"=u16 1003 ("左工位状态")) -> ()  [unwired: 9 in, 1 out]
                        n255 = for {
                          N: 12 -> [_]
                          tunnel: [cluster{dbl[], dbl[]} {[], []}] -> w260 mode=indexing
                        }
                        n256 = local write "右工位"(w260) -> ()
                        n257 = global read "Global.vi" "左启用"() -> (w258:i16)
                        n258 = case shown="1" w258 {
                          frame 0, Default {
                            n259 = global read "Global.vi" "Result"() -> (w269:refnum<vi>)
                            n260 = property class="Tbl"(reference=w269, "Row Headers[]"=string[] [] ("行首字符串[]"), "Value"=string[][] [] ("值"), "Active Cell"=T2 {"Row"=-2, "Column"=-2} ("活动单元格:活动单元格"), "Cell BG Color"=u32 16777216 ("活动单元格:单元格背景色")) -> ()  [unwired: 1 in, 2 out]
                          }
                          frame 1 {
                            n261 = global read "Global.vi" "Result  右工位"() -> (w274:refnum<vi>)
                            n262 = property class="Tbl"(reference=w274, "Row Headers[]"=string[] [] ("行首字符串[]"), "Value"=string[][] [] ("值"), "Active Cell"=T2 {"Row"=-2, "Column"=-2} ("活动单元格:活动单元格"), "Cell BG Color"=u32 16777216 ("活动单元格:单元格背景色")) -> ()  [unwired: 1 in, 2 out]
                          }
                        }
                      }
                    }
                  }
                  frame 1002 {
                    n263 = stacked-sequence {
                      frame #0 {
                        n264 = Wait (ms)(milliseconds to wait=u32 100 ("等待时间（毫秒）")) -> ()  [unwired: 1 out]
                        n265 = shared-variable "我的电脑\\Global.lvlib\\总成追溯码"() -> (w276:string)  [unwired: 1 in, 1 out]
                        n266 = shared-variable "我的电脑\\Global.lvlib\\传感器码-右"(w276) -> ()  [unwired: 1 in, 1 out]
                      }
                      frame #1 {
                        n267 = global read "Global1.vi" "联机模式"() -> (w278:enum16{"单机", "追溯"})
                        n268 = case shown="\"追溯\"" w278 {
                          selector: w278 -> [_ w288]
                          frame "单机", Default {
                          }
                          frame "追溯" {
                            n269 = shared-variable "我的电脑\\Global.lvlib\\传感器码-右"() -> (w279:string)  [unwired: 1 in, 1 out]
                            n270 = global read "追溯Global.vi" "PRODUCT_ID"() -> (w287:string)
                            n271 = Bundle("String"=w279, "PRODUCT_ID"=w287) -> (w285:cluster{"String":string, "PRODUCT_ID":string})  [unwired: 1 in]
                            n272 = call "GetSQLstring.vi"("联机模式"=w288) -> ("错误输出"=w284:errorcluster, "连接字符串"=w286:string)  [unwired: 9 in]
                            n273 = call-poly <vilib>:"DB Tools Open Connection.vi"("error in (no error)"=w284, "connection information"=w286) -> ("error out"=w281:errorcluster, "connection reference"=w283:T8)  [unwired: 6 in]
                            n274 = Build Array(w285) -> (w280:cluster{"String":string, "PRODUCT_ID":string}[])
                            n275 = for {
                              tunnel: w280 -> [w295] mode=indexing
                              tunnel: w283 -> [w294]
                              shift-right: [w290] -> w282
                              shift-left: w281 -> [w289]
                              n276 = call <vilib>:"DB Tools Insert Data.vi"("data"=w295, "error in (no error)"=w289, "columns"=string[] ["CODE_SENSOR", "PRODUCT_ID"], "table"="Code", "connection reference"=w294) -> ("error out"=w291:errorcluster)  [unwired: 5 in, 1 out]
                              n277 = case shown="无错误" w291 {
                                selector: w291 -> [w296 w297]
                                tunnel: [w296 w298] -> w290
                                frame No Error {
                                }
                                frame Error {
                                n278 = call <vilib>:"Clear Errors.vi"("error in (no error)"=w297) -> ("error out"=w298:errorcluster)  [unwired: 5 in, 1 out]
                                }
                              }
                            }
                            n279 = call <vilib>:"Simple Error Handler.vi"("error in (no error)"=w282) -> ()  [unwired: 4 in, 5 out]
                          }
                        }
                      }
                      frame #2 {
                        n280 = global read "Global1.vi" "联机模式"() -> (w299:enum16{"单机", "追溯"})
                        n281 = case shown="\"追溯\"" w299 {
                          selector: w299 -> [_ w320]
                          frame "单机", Default {
                          }
                          frame "追溯" {
                            w312 = "'"
                            n282 = shared-variable "我的电脑\\Global.lvlib\\传感器码-右"() -> (w302:string)  [unwired: 1 in, 1 out]
                            n283 = global read "追溯Global.vi" "PRODUCT_ID"() -> (w313:string)
                            n284 = call "GetSQLstring.vi"("联机模式"=w320) -> ("错误输出"=w318:errorcluster, "连接字符串"=w319:string)  [unwired: 9 in]
                            n285 = Concatenate Strings("SELECT CODE_ID FROM CODE  WHERE CODE_SENSOR = '" ("table"), w302, w312, " AND PRODUCT_ID='" ("字符串"), w313, w312) -> (w311:string)
                            n286 = call-poly <vilib>:"DB Tools Open Connection.vi"("error in (no error)"=w318, "connection information"=w319) -> ("error out"=w317:errorcluster, "connection reference"=w316:T8)  [unwired: 6 in]
                            n287 = call-poly <vilib>:"DB Tools Execute Query.vi"("error in (no error)"=w317, "SQL query"=w311, "connection reference"=w316) -> ("error out"=w310:errorcluster, "recordset reference"=w309:T9)  [unwired: 5 in]
                            n288 = call-poly <vilib>:"DB Tools Fetch Recordset Data.vi"("error in (no error)"=w310, "recordset reference"=w309) -> ("error out"=w308:errorcluster, "recordset data"=w307:variant[][])  [unwired: 3 in, 1 out]
                            n289 = Variant To Data(error in=w308, type=string[][] [], Variant=w307) -> (data=w305:string[][])  [unwired: 1 out]
                            n290 = Index Array(array=w305, index (row)=0 ("索引 (行)")) -> (element=w304:string[])  [unwired: 1 in]
                            n291 = Index Array(array=w304, index=0 ("索引")) -> (element=w303:string)
                            n292 = local write "右code 2"(w303) -> ()
                          }
                        }
                      }
                      frame #3 {
                        n293 = Wait (ms)(milliseconds to wait=u32 50 ("等待时间（毫秒）")) -> ()  [unwired: 1 out]
                        n294 = local write "STEP 2"("自动" ("STEP 2")) -> ()
                        n295 = call "右工位状态.vi"("枚举"=enum16{"Read", "Write"}."Write", "Status_Write"=u16 1003 ("左工位状态")) -> ()  [unwired: 9 in, 1 out]
                        n296 = for {
                          N: 12 -> [_]
                          tunnel: [cluster{dbl[], dbl[]} {[], []}] -> w323 mode=indexing
                        }
                        n297 = local write "右工位"(w323) -> ()
                        n298 = global read "Global.vi" "左启用"() -> (w321:i16)
                        n299 = case shown="1" w321 {
                          frame 0, Default {
                            n300 = global read "Global.vi" "Result"() -> (w332:refnum<vi>)
                            n301 = property class="Tbl"(reference=w332, "Row Headers[]"=string[] [] ("行首字符串[]"), "Value"=string[][] [] ("值"), "Active Cell"=T2 {"Row"=-2, "Column"=-2} ("活动单元格:活动单元格"), "Cell BG Color"=u32 16777216 ("活动单元格:单元格背景色")) -> ()  [unwired: 1 in, 2 out]
                          }
                          frame 1 {
                            n302 = global read "Global.vi" "Result  右工位"() -> (w337:refnum<vi>)
                            n303 = property class="Tbl"(reference=w337, "Row Headers[]"=string[] [] ("行首字符串[]"), "Value"=string[][] [] ("值"), "Active Cell"=T2 {"Row"=-2, "Column"=-2} ("活动单元格:活动单元格"), "Cell BG Color"=u32 16777216 ("活动单元格:单元格背景色")) -> ()  [unwired: 1 in, 2 out]
                          }
                        }
                      }
                    }
                  }
                }
              }
              frame "不合格" {
                n304 = Wait (ms)(milliseconds to wait=u32 100 ("等待时间（毫秒）")) -> ()  [unwired: 1 out]
                n305 = local write "STEP 2"("等待" ("STEP")) -> ()
              }
              frame "报表" {
                n306 = stacked-sequence {
                  frame #0 {
                    n307 = stacked-sequence {
                      seq-local: [w343 _ _] -> [_ w346 _]
                      frame #0 {
                        n308 = shared-variable "我的电脑\\Global.lvlib\\传感器码-右"() -> (w342:string)  [unwired: 1 in, 1 out]
                        n309 = call "Report1.vi"("文件重命名"=TRUE, "文件名称"=w342, "检测结果"="判定结果 2") -> ("PRODUCT_VAULE"=w343:string)  [unwired: 7 in, 1 out]
                      }
                      frame #1 {
                        n310 = global read "Global1.vi" "联机模式"() -> (w345:enum16{"单机", "追溯"})
                        n311 = case shown="\"追溯\"" w345 {
                          tunnel: w346 -> [_ w348]
                          frame "单机", Default {
                          }
                          frame "追溯" {
                            n312 = global read "Global.vi" "左启用"() -> (w347:i16)
                            n313 = case shown="0, 默认" w347 {
                              tunnel: [w357 w358] -> w355
                              frame 0, Default {
                                n314 = global read "Global.vi" "Result"() -> (w357:refnum<vi>)
                              }
                              frame 1 {
                                n315 = global read "Global.vi" "Result  右工位"() -> (w358:refnum<vi>)
                              }
                            }
                            n316 = property class="Tbl"(reference=w355) -> (reference out=w354:refnum<vi>, "Row Headers[]"=w352:string[])  [unwired: 1 in, 1 out]
                            n317 = property class="Tbl"(reference=w354) -> ("Value"=w353:string[][])  [unwired: 1 in, 2 out]
                            n318 = for {
                              tunnel: w353 -> [w361] mode=indexing
                              tunnel: w352 -> [w362] mode=indexing
                              tunnel: [w359] -> w349 mode=indexing if=w360
                              n319 = Build Array (concatenate)(w362, w361) -> (w359:string[])
                              n320 = Index Array(array=w361) -> (element=w363:string)  [unwired: 1 in]
                              n321 = case shown="默认" w363 {
                                tunnel: [TRUE FALSE] -> w360
                                frame Default {
                                }
                                frame "" {
                                }
                              }
                            }
                            n322 = global read "追溯Global.vi" "DEVICE_ID"() -> (w351:string)
                            n323 = global read "追溯Global.vi" "USER_ID"() -> (w356:string)
                            n324 = local read "右code 2"() -> (w350:string)
                            n325 = call "UPRESULT - 副本.vi"("DEVICE_ID"=w351, "USER_ID"=w356, "CODE_ID"=w350, "RESULT_VALUE"=w348) -> ()  [unwired: 11 in, 1 out]
                            n326 = call "UPTEST - 副本.vi"("Result"=w349, "CODE_ID"=w350, "DEVICE_ID"=w351) -> ()  [unwired: 6 in, 1 out]
                          }
                        }
                      }
                      frame #2 {
                        n327 = local write "STEP 2"("自动" ("STEP 2")) -> ()
                      }
                    }
                  }
                  frame #1 {
                    n328 = global write "Global.vi" "计时开始"(FALSE ("计时开始")) -> ()
                    n329 = call "右工位状态.vi"("枚举"=enum16{"Read", "Write"}."Write", "Status_Write"=i16 3) -> ()  [unwired: 9 in, 1 out]
                  }
                  frame #2 {
                    n330 = local write "STEP"("进入自动" ("STEP")) -> ()
                    n331 = global write "Global.vi" "计时开始"(FALSE ("计时开始")) -> ()
                  }
                }
              }
            }
            n332 = global read "Global.vi" "程序关闭"() -> (w12:bool)
            "STEP 3" <- "STEP 2"
          }
        }
        frame Enabled {
        }
      }
      n333 = while {
        stop <- w374 stop-if-true
        n334 = Wait Until Next ms Multiple(millisecond multiple=u32 2 ("毫秒倍数")) -> ()  [unwired: 1 out]
        n335 = case shown="\"报表\"" "STEP" {
          frame "等待", Default {
            n336 = Wait (ms)(milliseconds to wait=u32 200 ("等待时间（毫秒）")) -> ()  [unwired: 1 out]
            n337 = local write "STEP"("自动" ("STEP")) -> ()
          }
          frame "手动" {
          }
          frame "退出自动" {
            w378 = enum16{"Read", "Write"}."Write" ("枚举")
            n338 = global write "Global.vi" "计时开始"(FALSE ("计时开始")) -> ()
            n339 = local write "STEP"("等待" ("STEP")) -> ()
            n340 = call "设备状态.vi"("枚举"=w378, "Status_Write"=i16 0) -> ()  [unwired: 9 in, 1 out]
            n341 = call "跳转步骤.vi"("枚举"=w378, "Status_Write"=i16 1001) -> ()  [unwired: 9 in, 1 out]
          }
          frame "进入自动" {
            n342 = global read "Global.vi" "程序自动"() -> (w383:refnum<vi>)
            n343 = local write "STEP"("自动" ("STEP")) -> ()
            n344 = property class="Bool"(reference=w383, "Value"=TRUE) -> ()  [unwired: 1 in, 2 out]
          }
          frame "扫码" {
            n345 = stacked-sequence {
              frame #0 {
                w386 = "请扫传感器码！" ("提示信息")
                n346 = call "浮动通知.vi"("通知内容"=w386) -> ()  [unwired: 11 in]
                n347 = call "输入框.vi"("提示信息"=w386) -> ("条形码输出"=w387:string)
                n348 = case shown="默认" w387 {
                  selector: w387 -> [w388 _]
                  tunnel: [w390 "退出自动" ("State(s) in Front (\"\")")] -> w385
                  frame Default {
                    n349 = shared-variable "我的电脑\\Global.lvlib\\工位追溯码"(w388) -> ()  [unwired: 1 in, 1 out]
                    n350 = global read "Global1.vi" "联机模式"() -> (w389:enum16{"单机", "追溯"})
                    n351 = case shown="\"单机\", 默认" w389 {
                      tunnel: ["自动" ("State(s) in Front (\"\")") w396] -> w390
                      tunnel: w388 -> [_ w395]
                      frame "单机", Default {
                      }
                      frame "追溯" {
                        n352 = call "Get_CODE_ID.vi"("CODE_MAIN"=w395) -> ("CODE_ID"=w392:string)  [unwired: 10 in]
                        n353 = global write "追溯Global.vi" "CODE_ID"(w392) -> ()
                        n354 = global read "追溯Global.vi" "PRODUCT_ID"() -> (w394:string)
                        n355 = call "GET_PRESTATUS.vi"("CODE_ID"=w392, "PRODUCT_ID"=w394) -> ("OK?"=w393:bool)  [unwired: 8 in, 1 out]
                        n356 = case shown="真" w393 {
                          tunnel: [w400 "自动" ("State(s) in Front (\"\")")] -> w396
                          frame False {
                            n357 = global read "追溯Global.vi" "前序设备ID"() -> (w399:string)
                            n358 = Equal?(x=w399, y="") -> (x = y?=w398:bool)
                            n359 = case shown="真" w398 {
                              tunnel: ["退出自动" ("State(s) in Front (\"\")") "自动" ("State(s) in Front (\"\")")] -> w400
                              frame False {
                                n360 = global read "Global.vi" "上序状态"() -> (w403:refnum<vi>)
                                n361 = One Button Dialog(message="前序工位检测不合格！" ("消息")) -> ()  [unwired: 1 in, 1 out]
                                n362 = property class="Str"(reference=w403, "Text.BGColor"=u32 16711680 ("文本.文本颜色:背景色"), "Text.Text"="不合格" ("文本.文本")) -> ()  [unwired: 1 in, 2 out]
                              }
                              frame True {
                                n363 = global read "Global.vi" "上序状态"() -> (w408:refnum<vi>)
                                n364 = property class="Str"(reference=w408, "Text.BGColor"=u32 6618880 ("文本.文本颜色:背景色"), "Text.Text"="首序" ("文本.文本")) -> ()  [unwired: 1 in, 2 out]
                              }
                            }
                          }
                          frame True {
                            n365 = global read "Global.vi" "生产数量"() -> (w413:i32)
                            n366 = global read "Global.vi" "上序状态"() -> (w412:refnum<vi>)
                            n367 = Increment(x=w413) -> (x+1=w414:i32)
                            n368 = property class="Str"(reference=w412, "Text.BGColor"=u32 6618880 ("文本.文本颜色:背景色"), "Text.Text"="合格" ("文本.文本")) -> ()  [unwired: 1 in, 2 out]
                            n369 = global write "Global.vi" "生产数量"(w414) -> ()
                          }
                        }
                      }
                    }
                  }
                  frame "", "exit" {
                  }
                }
                n370 = local write "STEP"(w385) -> ()
              }
              frame #1 {
                n371 = Wait (ms)(milliseconds to wait=u32 200 ("等待时间（毫秒）")) -> ()  [unwired: 1 out]
              }
            }
          }
          frame "工位判断" {
          }
          frame "初始化" {
            n372 = stacked-sequence {
              frame #0 {
                n373 = global write "Global.vi" "IO_Stop"(TRUE ("IO_Stop")) -> ()
                n374 = global write "Global.vi" "计时开始"(FALSE ("计时开始")) -> ()
                n375 = local write "判定结果"(bool[][] [] ("判定结果")) -> ()
              }
              frame #1 {
                n376 = for {
                  N: 12 -> [_]
                  tunnel: [cluster{dbl[], dbl[]} {[], []}] -> w421 mode=indexing
                }
                n377 = local write "左工位"(w421) -> ()
              }
              frame #2 {
                w424 = -2 ("维数大小")
                n378 = global read "Global.vi" "Result"() -> (w433:refnum<vi>)
                n379 = Initialize Array(TRUE, 12 ("维数大小")) -> (→"初始化":bool[])
                n380 = property class="Tbl"(reference=w433, "Value"=string[][] []) -> (reference out=w434:refnum<vi>, error out=w435:errorcluster)  [unwired: 1 in]
                n381 = property class="Tbl"(reference=w434, error in=w435, "Row Headers[]"=string[] [] ("列首字符串[]")) -> (reference out=w427:refnum<vi>)  [unwired: 1 out]
                n382 = Bundle("维数大小"=w424, "维数大小"=w424) -> (w425:cluster{"维数大小":i32, "维数大小":i32})  [unwired: 1 in]
                n383 = property class="Tbl"(reference=w427, "Active Cell"=w425, "Cell BG Color"=u32 16777216 ("活动单元格:单元格背景色")) -> ()  [unwired: 1 in, 2 out]
              }
              frame #3 {
                n384 = local write "STEP"("自动" ("STEP")) -> ()
              }
            }
          }
          frame "判定" {
            n385 = stacked-sequence {
              frame #0 {
                n386 = global read "A131258.vi" "结果判定参数"() -> (w438:T5)
                n387 = global read "Global.vi" "Result"() -> (w440:refnum<vi>)
                n388 = local read "左工位"() -> (w439:cluster{dbl[], dbl[]}[])
                n389 = call "试验判定.vi"("Result"=w440, "判定参数"=w438, "XY曲线"=w439) -> ("判定项长度"=w437:i32, "OK？"=w441:bool)  [unwired: 7 in]
                n390 = case shown="真" w441 {
                  frame False {
                    n391 = call "左工位结果.vi"("枚举"=enum16{"Read", "Write"}."Write", "Status_Write"=u16 2 ("左工位生产结果")) -> ()  [unwired: 9 in, 1 out]
                  }
                  frame True {
                    n392 = call "左工位结果.vi"("枚举"=enum16{"Read", "Write"}."Write", "Status_Write"=u16 1 ("左工位生产结果")) -> ()  [unwired: 9 in, 1 out]
                  }
                }
                n393 = global write "判定参数.vi" "左判定长度"(w437) -> ()
                n394 = Build Array(TRUE ("元素"), w441) -> (w444:bool[])
                n395 = local read "判定结果"() -> (w445:bool[][])
                n396 = Build Array(w444) -> (w443:bool[][])
                n397 = Build Array (concatenate)(w445, w443) -> (w446:bool[][])
                n398 = local write "判定结果"(w446) -> ()
              }
              frame #1 {
                n399 = local write "STEP"("报表" ("STEP")) -> ()
                n400 = call "左工位状态.vi"("枚举"=enum16{"Read", "Write"}."Write", "Status_Write"=i16 660) -> ()  [unwired: 9 in, 1 out]
              }
            }
          }
          frame "自动" {
            n401 = global read "Global.vi" "左状态"() -> (w454:i16)
            n402 = case shown="600" w454 {
              frame 0, Default {
              }
              frame 1 {
              }
              frame 3 {
                n403 = stacked-sequence {
                  frame #0 {
                    n404 = call "左工位结果.vi"("枚举"=enum16{"Read", "Write"}."Write", "Status_Write"=i16 0) -> ()  [unwired: 9 in, 1 out]
                  }
                  frame #1 {
                    n405 = global read "Global.vi" "空载速度(°/s) 2"() -> (w457:sgl)
                    n406 = Multiply(x=w457, y=sgl 6.0) -> (x*y=w458:sgl)
                    n407 = global write "Global.vi" "空载速度(°/s)"(w458) -> ()
                  }
                }
              }
              frame 200 {
                n408 = stacked-sequence {
                  frame #0 {
                    w468 = TRUE ("Initialize 2")
                    n409 = local write "Initialize 2"(w468) -> ()
                    n410 = local write "Initialize 4"(w468) -> ()
                    n411 = call "左工位结果.vi"("枚举"=enum16{"Read", "Write"}."Write", "Status_Write"=u16 0 ("左工位生产结果")) -> ()  [unwired: 9 in, 1 out]
                    n412 = local write "判定结果"(bool[][] [] ("判定结果")) -> ()
                    n413 = for {
                      N: 4 -> [_]
                      tunnel: [cluster{dbl[], dbl[]} {[], []}] -> w466 mode=indexing
                    }
                    n414 = global read "Global.vi" "Result"() -> (w461:refnum<vi>)
                    n415 = local write "左工位"(w466) -> ()
                    n416 = property class="Tbl"(reference=w461, "Row Headers[]"=string[] [] ("行首字符串[]"), "Value"=string[][] [] ("值"), "Active Cell"=T2 {"Row"=-2, "Column"=-2} ("活动单元格:活动单元格"), "Cell BG Color"=u32 16777216 ("活动单元格:单元格背景色")) -> ()  [unwired: 1 in, 2 out]
                  }
                  frame #1 {
                    n417 = local read "左工位"() -> (w472:cluster{dbl[], dbl[]}[])
                    n418 = for {
                      tunnel: [w475] -> w473 mode=indexing
                      tunnel: w472 -> [w474] mode=indexing
                      i -> [w476]
                      n419 = case shown="1" w476 {
                        tunnel: [w477 w478 w486] -> w475
                        tunnel: w474 -> [w477 _ _]
                        frame Default {
                        }
                        frame 0 {
                          n420 = global read "A131258.vi" "判定框参数"() -> (w483:T6)
                          n421 = Unbundle By Name(w483) -> ("正向判定X值.下限"=w482:dbl, "正向判定X值.上限"=w481:dbl, "正向判定Y值.下限"=w480:dbl, "正向判定Y值.上限"=w479:dbl)
                          n422 = Build Array(w481, w481, w482, w482, w481) -> (w485:dbl[])
                          n423 = Build Array(w479, w480, w480, w479, w479) -> (w484:dbl[])
                          n424 = Bundle(w485, w484) -> (w478:cluster{dbl[], dbl[]})  [unwired: 1 in]
                        }
                        frame 1 {
                          n425 = global read "A131258.vi" "判定框参数"() -> (w491:T6)
                          n426 = Unbundle By Name(w491) -> ("逆向判定X值.下限"=w490:dbl, "逆向判定X值.上限"=w489:dbl, "逆向判定Y值.下限"=w488:dbl, "逆向判定Y值.上限"=w487:dbl)
                          n427 = Build Array(w489, w489, w490, w490, w489) -> (w493:dbl[])
                          n428 = Build Array(w487, w488, w488, w487, w487) -> (w492:dbl[])
                          n429 = Bundle(w493, w492) -> (w486:cluster{dbl[], dbl[]})  [unwired: 1 in]
                        }
                      }
                    }
                    n430 = local write "左工位"(w473) -> ()
                  }
                  frame #2 {
                    n431 = call "左工位状态.vi"("枚举"=enum16{"Read", "Write"}."Write", "Status_Write"=i16 500) -> ()  [unwired: 9 in, 1 out]
                  }
                }
              }
              frame 500 {
                n432 = local read "左工位"() -> (w497:cluster{dbl[], dbl[]}[])
                n433 = for {
                  tunnel: w497 -> [w499] mode=indexing
                  tunnel: [w498] -> w496 mode=indexing
                  i -> [w500]
                  n434 = case shown="2" w500 {
                    tunnel: w499 -> [w501 w524]
                    tunnel: [w501 w515] -> w498
                    frame Default {
                    }
                    frame 2 {
                      n435 = global read "全局1.vi" "左加载"() -> (w510:dbl)
                      n436 = global read "A131258.vi" "系数"() -> (w511:T7)
                      n437 = local write "Initialize 2"(FALSE ("Initialize 2")) -> ()
                      n438 = Unbundle By Name(w511) -> ("左零点漂移.正"=w509:dbl, "左空载.正转"=w508:dbl)
                      n439 = case shown="真" "Initialize 2" {
                        tunnel: [w529 0.0] -> w520
                        frame False {
                          n440 = global read "全局 1.vi" "工位2正向磨合开始时间"() -> (w533:u32)
                          n441 = Tick Count (ms)() -> (millisecond timer value=w532:u32)
                          n442 = Subtract(x=w532, y=w533) -> (x-y=w531:u32)
                          n443 = Divide(x=w531, y=u32 1000) -> (x/y=w529:dbl)
                          n444 = global write "全局 1.vi" "工位2正向磨合结束时间"(w529) -> ()
                        }
                        frame True {
                          n445 = Tick Count (ms)() -> (millisecond timer value=w534:u32)
                          n446 = global write "全局 1.vi" "工位2正向磨合开始时间"(w534) -> ()
                        }
                      }
                      n447 = Subtract(x=w510, y=w509) -> (x-y=w507:dbl)
                      n448 = Unbundle(w524) -> (w517:dbl[], w523:dbl[])
                      n449 = Multiply(x=w507, y=w508) -> (x*y=w503:dbl)
                      n450 = global read "A131258.vi" "工位滤波"() -> (w506:cluster{"启用滤波":bool, "滤波系数":dbl})
                      n451 = Unbundle By Name(w506) -> ("启用滤波"=w505:bool, "滤波系数"=w502:dbl)
                      n452 = case shown="真" w505 {
                        tunnel: [w525 w527] -> w504
                        tunnel: w503 -> [w525 w528]
                        tunnel: w502 -> [_ w526]
                        frame False {
                        }
                        frame True {
                          n453 = call-poly <userlib>:"MGI Running Average.vi"("Averaging Size"=w526, "Value"=w528) -> ("Average"=w527:dbl)  [unwired: 9 in]
                        }
                      }
                      n454 = Build Array (concatenate)(w523, w504) -> (w514:dbl[])
                      n455 = global read "Global.vi" "空载速度(°/s)"() -> (w519:sgl)
                      n456 = Divide(x=w520, y=1.0) -> (x/y=w513:dbl)
                      n457 = Multiply(x=w519, y=w513) -> (x*y=w518:dbl)
                      n458 = Build Array (concatenate)(w517, w518) -> (w516:dbl[])
                      n459 = Bundle(w516, w514) -> (w515:cluster{dbl[], dbl[]})  [unwired: 1 in]
                    }
                  }
                }
                n460 = local write "左工位"(w496) -> ()
              }
              frame 600 {
                n461 = local read "左工位"() -> (w537:cluster{dbl[], dbl[]}[])
                n462 = for {
                  tunnel: w537 -> [w539] mode=indexing
                  tunnel: [w538] -> w536 mode=indexing
                  i -> [w540]
                  n463 = case shown="0, 默认" w540 {
                    tunnel: w539 -> [w541 w564]
                    tunnel: [w541 w555] -> w538
                    frame 0, Default {
                    }
                    frame 3 {
                      n464 = global read "全局1.vi" "左加载"() -> (w550:dbl)
                      n465 = global read "A131258.vi" "系数"() -> (w551:T7)
                      n466 = local write "Initialize 4"(FALSE ("Initialize 2")) -> ()
                      n467 = Unbundle By Name(w551) -> ("左零点漂移.反"=w549:dbl, "左空载.反转"=w547:dbl)
                      n468 = case shown="假" "Initialize 4" {
                        tunnel: [w569 w576] -> w561
                        frame False {
                          n469 = global read "全局 1.vi" "工位2逆向磨合开始时间"() -> (w575:u32)
                          n470 = Tick Count (ms)() -> (millisecond timer value=w574:u32)
                          n471 = Subtract(x=w574, y=w575) -> (x-y=w573:u32)
                          n472 = global read "全局 1.vi" "工位2正向磨合结束时间"() -> (w571:dbl)
                          n473 = Divide(x=w573, y=u32 1000) -> (x/y=w570:dbl)
                          n474 = Subtract(x=w571, y=w570) -> (x-y=w569:dbl)
                        }
                        frame True {
                          n475 = Tick Count (ms)() -> (millisecond timer value=w577:u32)
                          n476 = global write "全局 1.vi" "工位2逆向磨合开始时间"(w577) -> ()
                          n477 = global read "全局 1.vi" "工位2正向磨合结束时间"() -> (w576:dbl)
                        }
                      }
                      n478 = Subtract(x=w550, y=w549) -> (x-y=w548:dbl)
                      n479 = Unbundle(w564) -> (w558:dbl[], w563:dbl[])
                      n480 = Multiply(x=w548, y=w547) -> (x*y=w544:dbl)
                      n481 = global read "A131258.vi" "工位滤波"() -> (w546:cluster{"启用滤波":bool, "滤波系数":dbl})
                      n482 = Unbundle By Name(w546) -> ("启用滤波"=w545:bool, "滤波系数"=w542:dbl)
                      n483 = case shown="真" w545 {
                        tunnel: w544 -> [w565 w568]
                        tunnel: [w565 w567] -> w543
                        tunnel: w542 -> [_ w566]
                        frame False {
                        }
                        frame True {
                          n484 = call-poly <userlib>:"MGI Running Average.vi"("Averaging Size"=w566, "Value"=w568) -> ("Average"=w567:dbl)  [unwired: 9 in]
                        }
                      }
                      n485 = Build Array (concatenate)(w563, w543) -> (w556:dbl[])
                      n486 = global read "Global.vi" "空载速度(°/s)"() -> (w560:sgl)
                      n487 = Divide(x=w561, y=1.0) -> (x/y=w553:dbl)
                      n488 = Multiply(x=w560, y=w553) -> (x*y=w559:dbl)
                      n489 = Build Array (concatenate)(w558, w559) -> (w557:dbl[])
                      n490 = Bundle(w557, w556) -> (w555:cluster{dbl[], dbl[]})  [unwired: 1 in]
                    }
                  }
                }
                n491 = local write "左工位"(w536) -> ()
              }
              frame 650 {
                n492 = local write "STEP"("判定" ("STEP")) -> ()
              }
              frame 1001 {
                n493 = stacked-sequence {
                  frame #0 {
                    n494 = Wait (ms)(milliseconds to wait=u32 50 ("等待时间（毫秒）")) -> ()  [unwired: 1 out]
                    n495 = shared-variable "我的电脑\\Global.lvlib\\工位追溯码"() -> (w579:string)  [unwired: 1 in, 1 out]
                    n496 = shared-variable "我的电脑\\Global.lvlib\\传感器码-左"(w579) -> ()  [unwired: 1 in, 1 out]
                  }
                  frame #1 {
                    n497 = global read "Global1.vi" "联机模式"() -> (w581:enum16{"单机", "追溯"})
                    n498 = case shown="\"单机\", 默认" w581 {
                      selector: w581 -> [_ w591]
                      frame "单机", Default {
                      }
                      frame "追溯" {
                        n499 = shared-variable "我的电脑\\Global.lvlib\\传感器码-左"() -> (w582:string)  [unwired: 1 in, 1 out]
                        n500 = global read "追溯Global.vi" "PRODUCT_ID"() -> (w588:string)
                        n501 = Bundle("String"=w582, "PRODUCT_ID"=w588) -> (w587:cluster{"String":string, "PRODUCT_ID":string})  [unwired: 1 in]
                        n502 = call "GetSQLstring.vi"("联机模式"=w591) -> ("错误输出"=w589:errorcluster, "连接字符串"=w590:string)  [unwired: 9 in]
                        n503 = call-poly <vilib>:"DB Tools Open Connection.vi"("error in (no error)"=w589, "connection information"=w590) -> ("error out"=w585:errorcluster, "connection reference"=w586:T8)  [unwired: 6 in]
                        n504 = Build Array(w587) -> (w583:cluster{"String":string, "PRODUCT_ID":string}[])
                        n505 = for {
                          tunnel: w586 -> [w599]
                          shift-right: [w596] -> w584
                          shift-left: w585 -> [w598]
                          tunnel: w583 -> [w592] mode=indexing
                          n506 = call <vilib>:"DB Tools Insert Data.vi"("data"=w592, "error in (no error)"=w598, "columns"=string[] ["CODE_SENSOR", "PRODUCT_ID"], "table"="Code", "connection reference"=w599) -> ("error out"=w597:errorcluster, "connection reference out"=w595:T8)  [unwired: 5 in]
                          n507 = case shown="错误 .." w597 {
                            selector: w597 -> [w601 w603]
                            tunnel: [w601 w604] -> w596
                            tunnel: [w600 w602] -> _
                            tunnel: w595 -> [w600 w602]
                            frame No Error {
                            }
                            frame Error {
                              n508 = call <vilib>:"Clear Errors.vi"("error in (no error)"=w603) -> ("error out"=w604:errorcluster)  [unwired: 5 in, 1 out]
                            }
                          }
                        }
                        n509 = call <vilib>:"Simple Error Handler.vi"("error in (no error)"=w584) -> ()  [unwired: 4 in, 5 out]
                      }
                    }
                  }
                  frame #2 {
                    n510 = global read "Global1.vi" "联机模式"() -> (w605:enum16{"单机", "追溯"})
                    n511 = case shown="\"单机\", 默认" w605 {
                      selector: w605 -> [_ w626]
                      frame "单机", Default {
                      }
                      frame "追溯" {
                        w618 = "'"
                        n512 = shared-variable "我的电脑\\Global.lvlib\\传感器码-左"() -> (w606:string)  [unwired: 1 in, 1 out]
                        n513 = global read "追溯Global.vi" "PRODUCT_ID"() -> (w619:string)
                        n514 = call "GetSQLstring.vi"("联机模式"=w626) -> ("错误输出"=w624:errorcluster, "连接字符串"=w625:string)  [unwired: 9 in]
                        n515 = Concatenate Strings("SELECT CODE_ID FROM CODE  WHERE CODE_SENSOR = '" ("table"), w606, w618, " AND PRODUCT_ID='" ("字符串"), w619, w618) -> (w617:string)
                        n516 = call-poly <vilib>:"DB Tools Open Connection.vi"("error in (no error)"=w624, "connection information"=w625) -> ("error out"=w623:errorcluster, "connection reference"=w622:T8)  [unwired: 6 in]
                        n517 = call-poly <vilib>:"DB Tools Execute Query.vi"("error in (no error)"=w623, "SQL query"=w617, "connection reference"=w622) -> ("error out"=w616:errorcluster, "recordset reference"=w615:T9)  [unwired: 5 in]
                        n518 = call-poly <vilib>:"DB Tools Fetch Recordset Data.vi"("error in (no error)"=w616, "recordset reference"=w615) -> ("error out"=w614:errorcluster, "recordset data"=w613:variant[][])  [unwired: 3 in, 1 out]
                        n519 = Variant To Data(error in=w614, type=string[][] [], Variant=w613) -> (data=w611:string[][])  [unwired: 1 out]
                        n520 = Index Array(array=w611, index (row)=0 ("索引 (行)")) -> (element=w610:string[])  [unwired: 1 in]
                        n521 = Index Array(array=w610, index=0 ("索引")) -> (element=→"左code":string)
                      }
                    }
                  }
                  frame #3 {
                    n522 = Wait (ms)(milliseconds to wait=u32 50 ("等待时间（毫秒）")) -> ()  [unwired: 1 out]
                    n523 = for {
                      N: 12 -> [_]
                      tunnel: [cluster{dbl[], dbl[]} {[], []}] -> w636 mode=indexing
                    }
                    n524 = global read "Global.vi" "Result"() -> (w634:refnum<vi>)
                    n525 = property class="Tbl"(reference=w634, "Row Headers[]"=string[] [] ("行首字符串[]"), "Value"=string[][] [] ("值"), "Active Cell"=T2 {"Row"=-2, "Column"=-2} ("活动单元格:活动单元格"), "Cell BG Color"=u32 16777216 ("活动单元格:单元格背景色")) -> ()  [unwired: 1 in, 2 out]
                    n526 = local write "左工位"(w636) -> ()
                    n527 = call "左工位状态.vi"("枚举"=enum16{"Read", "Write"}."Write", "Status_Write"=u16 1003 ("左工位状态")) -> ()  [unwired: 9 in, 1 out]
                    n528 = global write "Global.vi" "计时开始"(TRUE ("计时开始")) -> ()
                  }
                }
              }
              frame 1002 {
                n529 = stacked-sequence {
                  frame #0 {
                    n530 = Wait (ms)(milliseconds to wait=u32 100 ("等待时间（毫秒）")) -> ()  [unwired: 1 out]
                    n531 = shared-variable "我的电脑\\Global.lvlib\\总成追溯码"() -> (w639:string)  [unwired: 1 in, 1 out]
                    n532 = shared-variable "我的电脑\\Global.lvlib\\传感器码-左"(w639) -> ()  [unwired: 1 in, 1 out]
                  }
                  frame #1 {
                    n533 = global read "Global1.vi" "联机模式"() -> (w641:enum16{"单机", "追溯"})
                    n534 = case shown="\"追溯\"" w641 {
                      selector: w641 -> [_ w651]
                      frame "单机", Default {
                      }
                      frame "追溯" {
                        n535 = shared-variable "我的电脑\\Global.lvlib\\传感器码-左"() -> (w642:string)  [unwired: 1 in, 1 out]
                        n536 = global read "追溯Global.vi" "PRODUCT_ID"() -> (w650:string)
                        n537 = Bundle("String"=w642, "PRODUCT_ID"=w650) -> (w648:cluster{"String":string, "PRODUCT_ID":string})  [unwired: 1 in]
                        n538 = call "GetSQLstring.vi"("联机模式"=w651) -> ("错误输出"=w647:errorcluster, "连接字符串"=w649:string)  [unwired: 9 in]
                        n539 = call-poly <vilib>:"DB Tools Open Connection.vi"("error in (no error)"=w647, "connection information"=w649) -> ("error out"=w644:errorcluster, "connection reference"=w646:T8)  [unwired: 6 in]
                        n540 = Build Array(w648) -> (w643:cluster{"String":string, "PRODUCT_ID":string}[])
                        n541 = for {
                          tunnel: w643 -> [w658] mode=indexing
                          tunnel: w646 -> [w657]
                          shift-right: [w653] -> w645
                          shift-left: w644 -> [w652]
                          n542 = call <vilib>:"DB Tools Insert Data.vi"("data"=w658, "error in (no error)"=w652, "columns"=string[] ["CODE_SENSOR", "PRODUCT_ID"], "table"="Code", "connection reference"=w657) -> ("error out"=w654:errorcluster)  [unwired: 5 in, 1 out]
                          n543 = case shown="无错误" w654 {
                            selector: w654 -> [w659 w660]
                            tunnel: [w659 w661] -> w653
                            frame No Error {
                            }
                            frame Error {
                              n544 = call <vilib>:"Clear Errors.vi"("error in (no error)"=w660) -> ("error out"=w661:errorcluster)  [unwired: 5 in, 1 out]
                            }
                          }
                        }
                        n545 = call <vilib>:"Simple Error Handler.vi"("error in (no error)"=w645) -> ()  [unwired: 4 in, 5 out]
                      }
                    }
                  }
                  frame #2 {
                    n546 = global read "Global1.vi" "联机模式"() -> (w662:enum16{"单机", "追溯"})
                    n547 = case shown="\"追溯\"" w662 {
                      selector: w662 -> [_ w683]
                      frame "单机", Default {
                      }
                      frame "追溯" {
                        w675 = "'"
                        n548 = shared-variable "我的电脑\\Global.lvlib\\传感器码-左"() -> (w663:string)  [unwired: 1 in, 1 out]
                        n549 = global read "追溯Global.vi" "PRODUCT_ID"() -> (w676:string)
                        n550 = call "GetSQLstring.vi"("联机模式"=w683) -> ("错误输出"=w681:errorcluster, "连接字符串"=w682:string)  [unwired: 9 in]
                        n551 = Concatenate Strings("SELECT CODE_ID FROM CODE  WHERE CODE_SENSOR = '" ("table"), w663, w675, " AND PRODUCT_ID='" ("字符串"), w676, w675) -> (w674:string)
                        n552 = call-poly <vilib>:"DB Tools Open Connection.vi"("error in (no error)"=w681, "connection information"=w682) -> ("error out"=w680:errorcluster, "connection reference"=w679:T8)  [unwired: 6 in]
                        n553 = call-poly <vilib>:"DB Tools Execute Query.vi"("error in (no error)"=w680, "SQL query"=w674, "connection reference"=w679) -> ("error out"=w673:errorcluster, "recordset reference"=w672:T9)  [unwired: 5 in]
                        n554 = call-poly <vilib>:"DB Tools Fetch Recordset Data.vi"("error in (no error)"=w673, "recordset reference"=w672) -> ("error out"=w671:errorcluster, "recordset data"=w670:variant[][])  [unwired: 3 in, 1 out]
                        n555 = Variant To Data(error in=w671, type=string[][] [], Variant=w670) -> (data=w668:string[][])  [unwired: 1 out]
                        n556 = Index Array(array=w668, index (row)=0 ("索引 (行)")) -> (element=w667:string[])  [unwired: 1 in]
                        n557 = Index Array(array=w667, index=0 ("索引")) -> (element=w666:string)
                        n558 = local write "左code"(w666) -> ()
                      }
                    }
                  }
                  frame #3 {
                    n559 = local write "STEP"("自动" ("STEP")) -> ()
                    n560 = for {
                      N: 12 -> [_]
                      tunnel: [cluster{dbl[], dbl[]} {[], []}] -> w690 mode=indexing
                    }
                    n561 = global read "Global.vi" "Result"() -> (w689:refnum<vi>)
                    n562 = call "左工位状态.vi"("枚举"=enum16{"Read", "Write"}."Write", "Status_Write"=u16 1003 ("左工位状态")) -> ()  [unwired: 9 in, 1 out]
                    n563 = property class="Tbl"(reference=w689, "Row Headers[]"=string[] [] ("行首字符串[]"), "Value"=string[][] [] ("值"), "Active Cell"=T2 {"Row"=-2, "Column"=-2} ("活动单元格:活动单元格"), "Cell BG Color"=u32 16777216 ("活动单元格:单元格背景色")) -> ()  [unwired: 1 in, 2 out]
                    n564 = local write "左工位"(w690) -> ()
                  }
                }
              }
            }
          }
          frame "不合格" {
            n565 = Wait (ms)(milliseconds to wait=u32 100 ("等待时间（毫秒）")) -> ()  [unwired: 1 out]
            n566 = local write "STEP"("等待" ("STEP")) -> ()
          }
          frame "报表" {
            n567 = global read "Global.vi" "左启用"() -> (w697:i16)
            n568 = case shown="1" w697 {
              frame 0, Default {
              }
              frame 1 {
                n569 = stacked-sequence {
                  frame #0 {
                    n570 = stacked-sequence {
                      seq-local: [w703 _ _] -> [_ w706 _]
                      frame #0 {
                        n571 = shared-variable "我的电脑\\Global.lvlib\\传感器码-左"() -> (w701:string)  [unwired: 1 in, 1 out]
                        n572 = call "时间秒.vi"() -> ("结果字符串"=w700:string)  [unwired: 11 in]
                        n573 = call <vilib>:"Space Constant.vi"() -> ("String"=w699:string)
                        n574 = Concatenate Strings(w701, w699, w700) -> (w698:string)
                        n575 = call "Report.vi"("文件重命名"=TRUE, "文件名称"=w698, "检测结果"="判定结果") -> ("PRODUCT_VAULE"=w703:string)  [unwired: 7 in, 1 out]
                      }
                      frame #1 {
                        n576 = global read "Global1.vi" "联机模式"() -> (w705:enum16{"单机", "追溯"})
                        n577 = case shown="\"追溯\"" w705 {
                          tunnel: w706 -> [_ w710]
                          frame "单机", Default {
                          }
                          frame "追溯" {
                            n578 = global read "Global.vi" "Result"() -> (w714:refnum<vi>)
                            n579 = property class="Tbl"(reference=w714) -> (reference out=w713:refnum<vi>, "Row Headers[]"=w711:string[])  [unwired: 1 in, 1 out]
                            n580 = property class="Tbl"(reference=w713) -> ("Value"=w712:string[][])  [unwired: 1 in, 2 out]
                            n581 = for {
                              tunnel: w712 -> [w718] mode=indexing
                              tunnel: w711 -> [w719] mode=indexing
                              tunnel: [w716] -> w708 mode=indexing if=w717
                              n582 = Build Array (concatenate)(w719, w718) -> (w716:string[])
                              n583 = Index Array(array=w718) -> (element=w720:string)  [unwired: 1 in]
                              n584 = case shown="\"\"" w720 {
                                tunnel: [TRUE FALSE] -> w717
                                frame Default {
                                }
                                frame "" {
                                }
                              }
                            }
                            n585 = global read "追溯Global.vi" "DEVICE_ID"() -> (w709:string)
                            n586 = global read "追溯Global.vi" "USER_ID"() -> (w715:string)
                            n587 = local read "左code"() -> (w707:string)
                            n588 = call "UPTEST.vi"("Result"=w708, "CODE_ID"=w707, "DEVICE_ID"=w709) -> ()  [unwired: 6 in, 1 out]
                            n589 = call "UPRESULT.vi"("DEVICE_ID"=w709, "USER_ID"=w715, "CODE_ID"=w707, "RESULT_VALUE"=w710) -> ()  [unwired: 11 in, 1 out]
                          }
                        }
                      }
                      frame #2 {
                        n590 = Wait (ms)(milliseconds to wait=u32 50 ("等待时间（毫秒）")) -> ()  [unwired: 1 out]
                      }
                    }
                  }
                  frame #1 {
                    n591 = call "设备状态.vi"("枚举"=enum16{"Read", "Write"}."Write", "Status_Write"=i16 5) -> ()  [unwired: 9 in, 1 out]
                  }
                  frame #2 {
                    n592 = global write "Global.vi" "计时开始"(FALSE ("计时开始")) -> ()
                    n593 = local write "STEP"("进入自动" ("STEP")) -> ()
                  }
                }
              }
            }
          }
        }
        n594 = global read "Global.vi" "程序关闭"() -> (w374:bool)
        "STEP 4" <- "STEP"
      }
    }
  }
